vi "ER2007 Test Panel Mock Up.vi"() -> ()   [LabVIEW 2013]
uses:
  Controls/Global ER2007.vi
panel:
  in  "Defeated":bool
  in  "Sim":bool
  in  "Radio Cell Selects":T1(ring)
  out "Clock":string
  in  "Reset DAQ":bool
  out "VPA Err":bool
  out "Elap-T":string="Lapsed Hrs"
  out "Last-T":string="Time"
  out "ProdVol":string="Produced Vol (cc)"
  out "Dnstrm-P":string="Downstrm P (psi)"
  out "Delta-P":string="Delta-P (psi)"
  out "Pore-P":string="Pore P (psi)"
  out "Conf-P":string="Confining P (psi)"
  out "TB":string="T-B (°C)"
  out "TA":string="T-A (°C)"
  out "FF23":string="FF 2-3"
  out "ER23":string="E-R 2-3 (Ohm-m)"
  out "ER14":string="E-R 1-4 (Ohm-m)"
  out "ER13":string="E-R 1-3 (Ohm-m)"
  out "ER12":string="E-R 1-2 (Ohm-m)"
  out "SampID":string="Sample ID"
  out "Frequency":string="Frequency (Hz)"
  out "Status":string="Status"
  out "Other PC Busy":bool
  out "GCD Reset":bool
  in  "TakePt":bool
  out "System Error":bool
  out "Refresh":bool
  out "SetupCell":i32
  out "GCDCell":i32
  out "SelCell":i32
  out "C5-Status":bool caption="VPA"
  out "C4-Status":bool caption="Manual"
  out "C3-Status":bool caption="VPA"
  out "C2-Status":bool caption="Manual"
  out "C1-Status":bool caption="Manual"
  in  "GCD Progress Titles":string="Initialize  Main Eng  Determ-R  Final Vals Close HP Close NAII"
  out "GCD Prog":bool[](array[boolean])
  out "Selected Data Cell":i32
  out "Cell Data Idx":i32
  out "Cur Time":dbl
  out "Schd Times":dbl[](array[numeric])
  out "GCD Err":bool
  out "GCD Busy":bool
  out "A/D Err":bool
  out "DAQ Run":bool
  in  "Utilities":bool
  out "F 2-3":dbl[](array[numeric])=[6.3872, 0.0, 5.0918, 5.4196, 0.0, 5.8365, 5.8365, 0.0] format="%.2f"
  out "Cell":string[](array[string])=["200", "2000", "20000", "200000", "2000000", "Cell 6B", "6B", "6C"]
  out "Copyrightl":string="Program ER2005, Version 1.00, DCI Inc, Copyright 2005, All Rights Reserved"
  in  "CurVals":bool
  in  "History":bool
  in  "Setup":bool
  in  "Stop":bool
  out "ER 2-3":dbl[](array[numeric])=[6.3872, 0.0, 5.0918, 5.4196, 0.0, 5.8365, 5.8365, 0.0] format="%.3f"
  out "ER 1-4":dbl[](array[numeric])=[6.1683, 0.0, 5.0447, 5.2485, 0.0, 5.6703, 5.6703, 0.0] format="%.3f"
  out "ER 1-3":dbl[](array[numeric])=[6.0887, 0.0, 4.9169, 5.2753, 0.0, 5.5338, 5.5338, 0.0] format="%.3f"
  out "ER 1-2":dbl[](array[numeric])=[6.7304, 0.0, 5.356, 5.9831, 0.0, 6.0646, 6.0646, 0.0] format="%.3f"
  out "Status":bool[](array[boolean])=[FALSE, FALSE, FALSE, FALSE, FALSE, FALSE, TRUE, FALSE]
  # "Test Data"
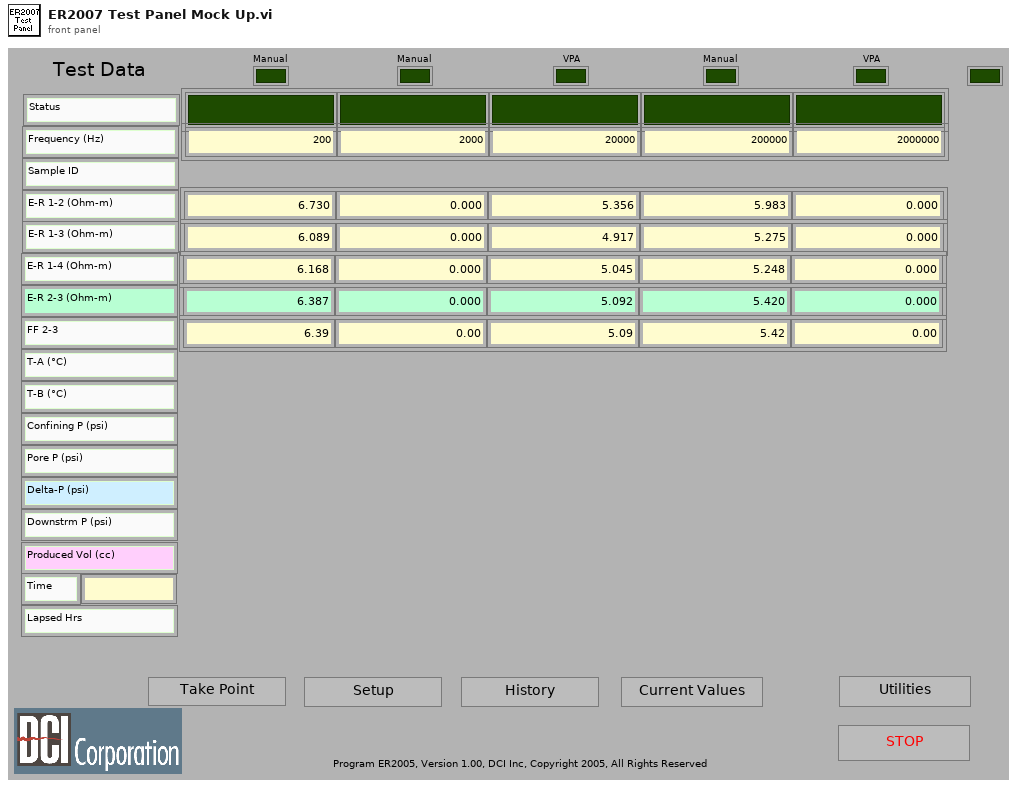
[diagram p1: front panel]
types:
  T1 = enum32{"No Selection", "CS 1", "CS 2", "CS 3", "CS 4", "CS 5", "CS 6"}
  T2 = cluster{"PageTitle":string, "NumLines":i32, "ChlNum":string[], "ChlDesc":string[], "ChlUnits":string[], "ChlZero":sgl[], "ChlFactor":sgl[], "ChlConfig":u16[]}[]
  T3 = enum16{"Cell 1", "Cell 2", "Cell 3", "Cell 4", "Cell 5", "Cell 6A", "Cell 6B", "Cell 6C"}[]
  T4 = cluster{"CurCell":i32, "Cell Data":cluster{"Cell ID":i32, "Cell Status":enum16{"Inactive", "Setup", "Active", "Done"}, "Project":string, "Sample #":string, "Rock Type":string, "Fluid Pair":string, "Rw":dbl, "Rw Temp":dbl, "Length":dbl, "Diameter":dbl, "Porosity":dbl, "Permeability":dbl, "4P":bool, "ElectSpace":dbl, "Frequency":dbl, "Amplitude":dbl, "DAQ Period":u32, "DAQ Units":u16, "Start Time":dbl, "Next Time":dbl, "Datafile":path, "Last Pore Vol":dbl, "Last Pore Xdcr":enum16{"<none>", "Lo Range", "Hi Range"}, "Last Resistor":enum16{"<none>", "Resistor 1", "Resistor 2", "Resistor 3", "Resistor 4", "Resistor 5", "Resistor 6"}, "CurData":dbl[][], "Comment":string}[]}
  T5 = cluster{"Cell ID":i32, "Cell Status":enum16{"Inactive", "Setup", "Active", "Done"}, "Project":string, "Sample #":string, "Rock Type":string, "Fluid Pair":string, "Rw":dbl, "Rw Temp":dbl, "Length":dbl, "Diameter":dbl, "Porosity":dbl, "Permeability":dbl, "4P":bool, "ElectSpace":dbl, "Frequency":dbl, "Amplitude":dbl, "DAQ Period":u32, "DAQ Units":u16, "Start Time":dbl, "Next Time":dbl, "Datafile":path, "Last Pore Vol":dbl, "Last Pore Xdcr":enum16{"<none>", "Lo Range", "Hi Range"}, "Last Resistor":enum16{"<none>", "Resistor 1", "Resistor 2", "Resistor 3", "Resistor 4", "Resistor 5", "Resistor 6"}, "CurData":dbl[][], "Comment":string}[]
  T6 = cluster{"Cell ID":i32, "Cell Status":enum16{"Inactive", "Setup", "Active", "Done"}, "Project":string, "Sample #":string, "Rock Type":string, "Fluid Pair":string, "Rw":dbl, "Rw Temp":dbl, "Length":dbl, "Diameter":dbl, "Porosity":dbl, "Permeability":dbl, "4P":bool, "ElectSpace":dbl, "Frequency":dbl, "Amplitude":dbl, "DAQ Period":u32, "DAQ Units":u16, "Start Time":dbl, "Next Time":dbl, "Datafile":path, "Last Pore Vol":dbl, "Last Pore Xdcr":enum16{"<none>", "Lo Range", "Hi Range"}, "Last Resistor":enum16{"<none>", "Resistor 1", "Resistor 2", "Resistor 3", "Resistor 4", "Resistor 5", "Resistor 6"}, "CurData":dbl[][], "Comment":string}
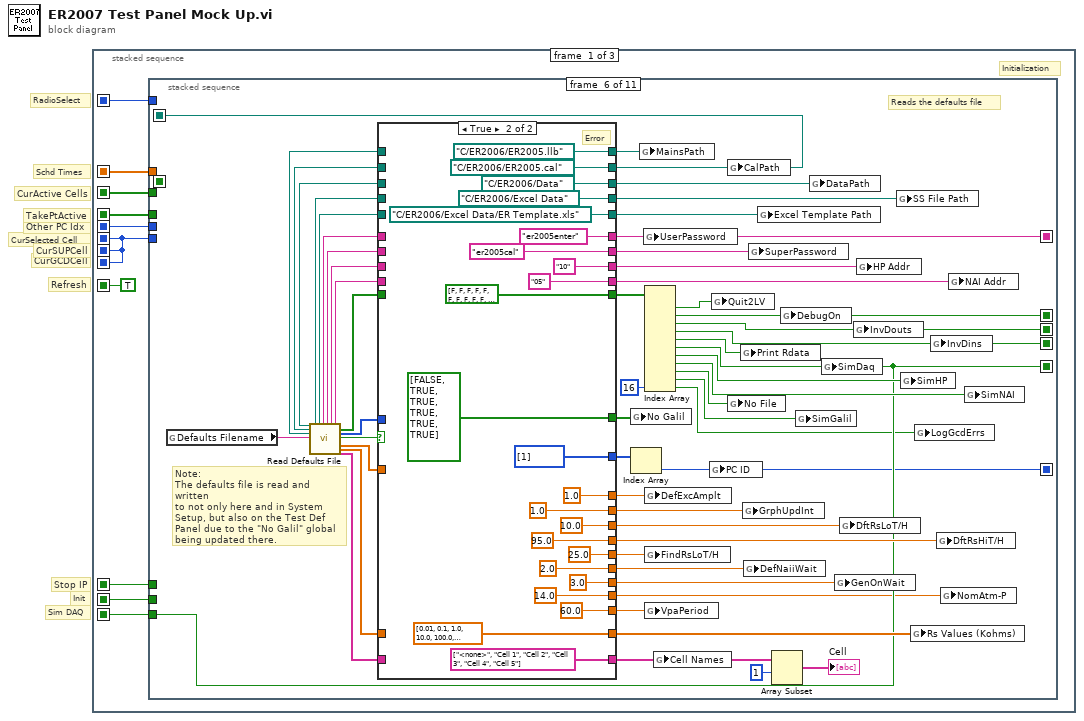
[diagram p0: block diagram]
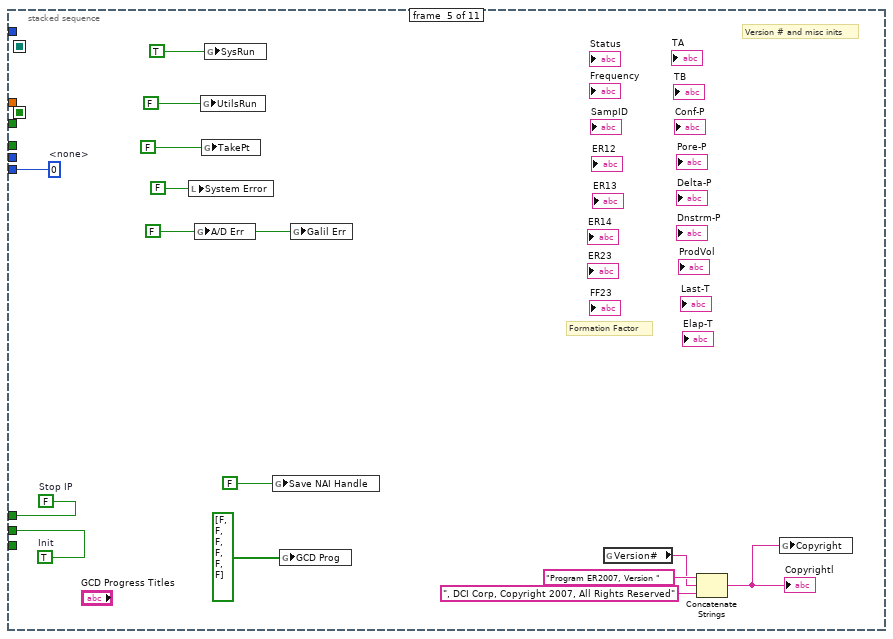
[diagram p6: hidden frame]
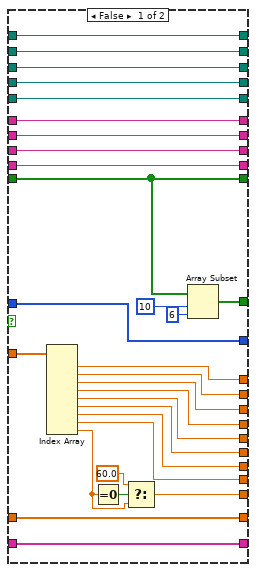
[diagram p7: hidden frame]
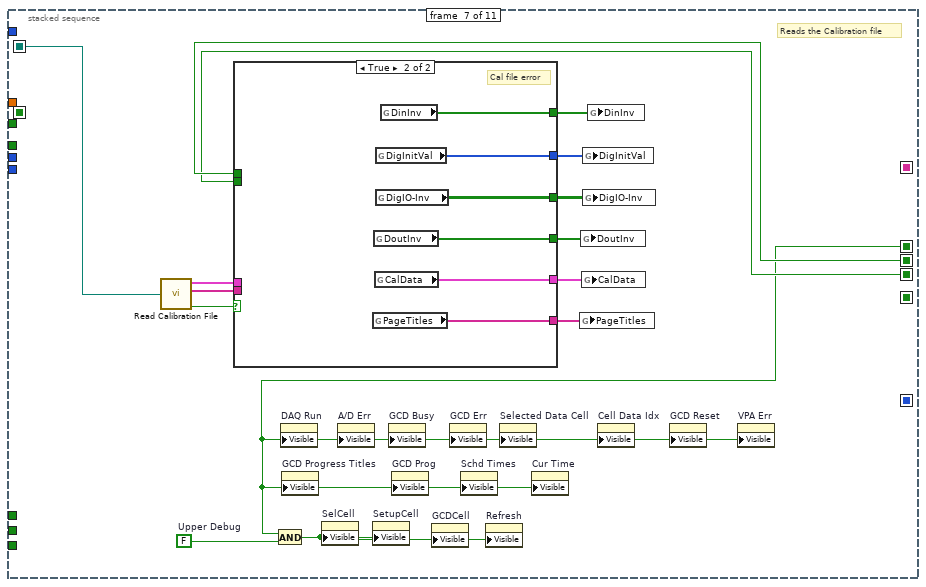
[diagram p8: hidden frame]
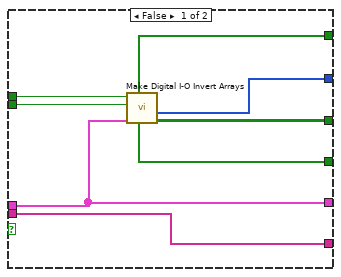
[diagram p9: hidden frame]
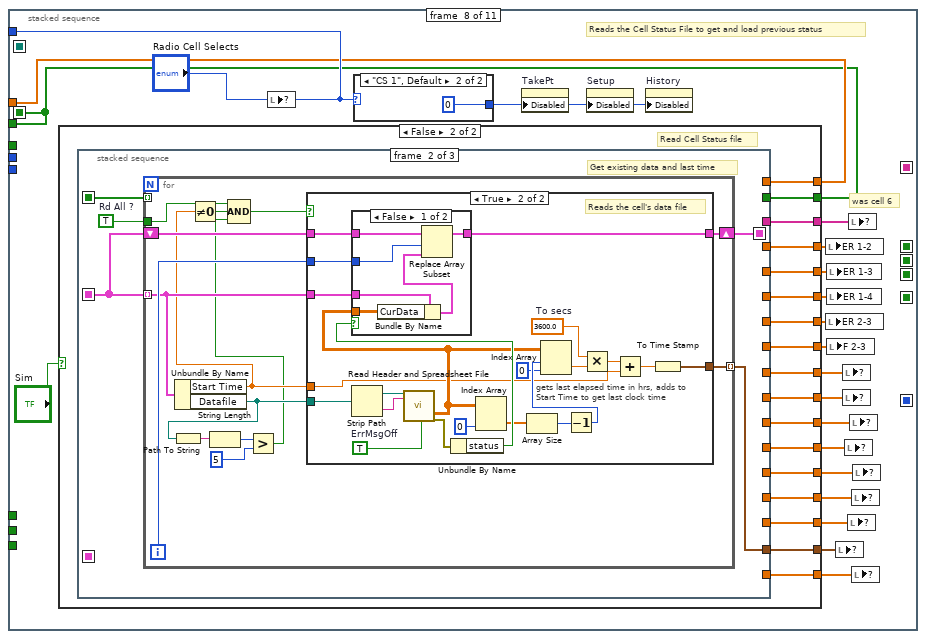
[diagram p10: hidden frame]
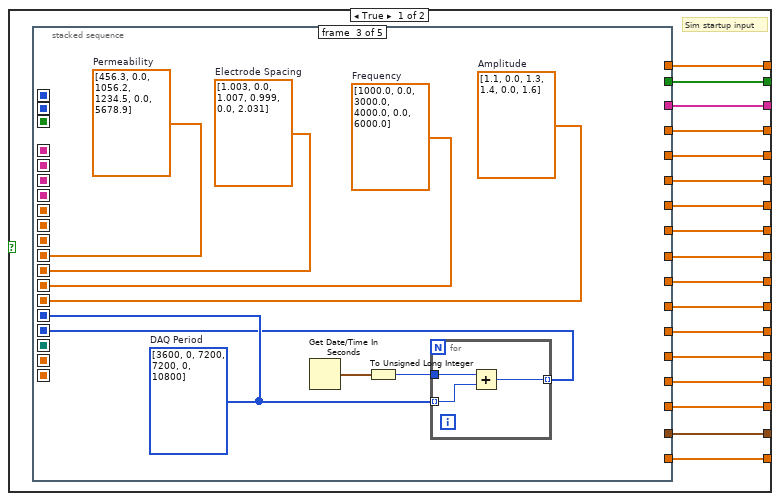
[diagram p11: hidden frame]
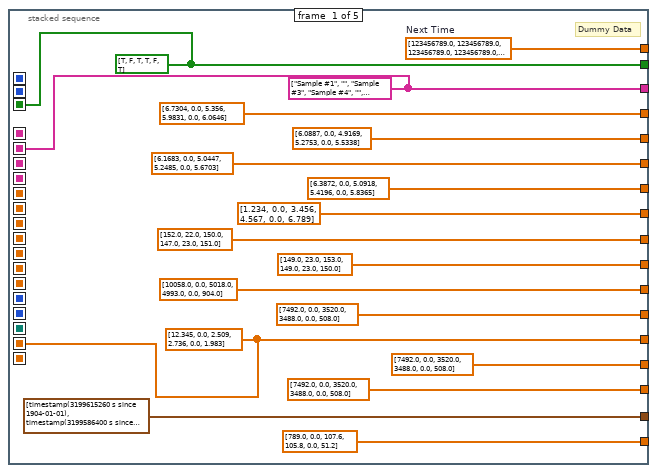
[diagram p12: hidden frame]
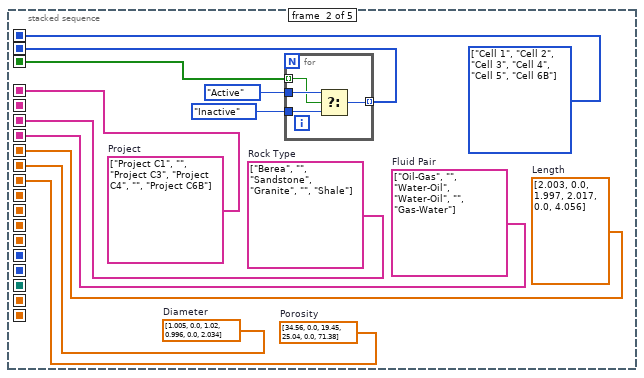
[diagram p13: hidden frame]
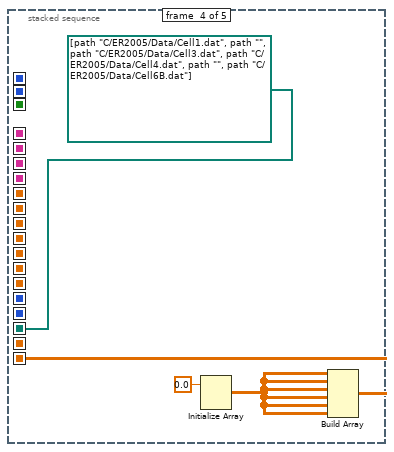
[diagram p14: hidden frame]
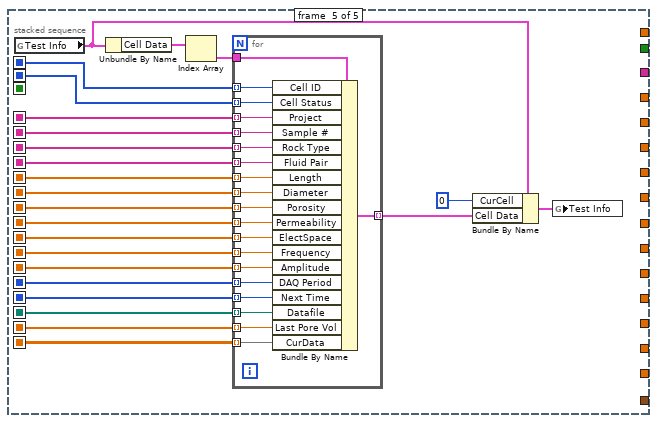
[diagram p15: hidden frame]
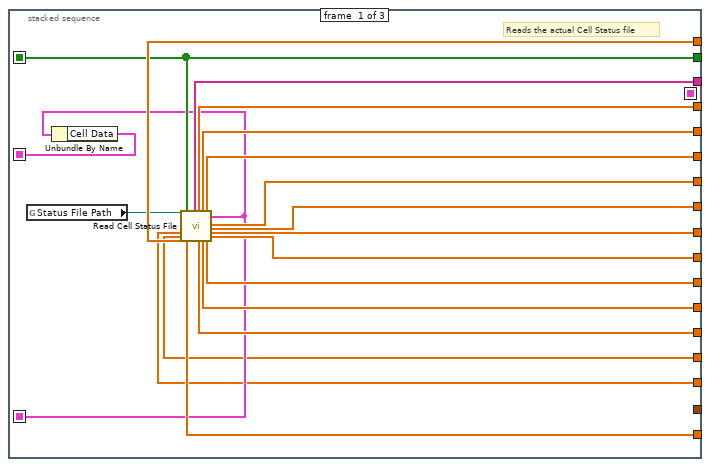
[diagram p16: hidden frame]
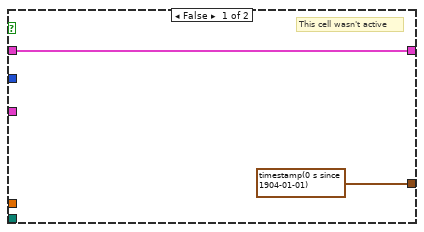
[diagram p17: hidden frame]
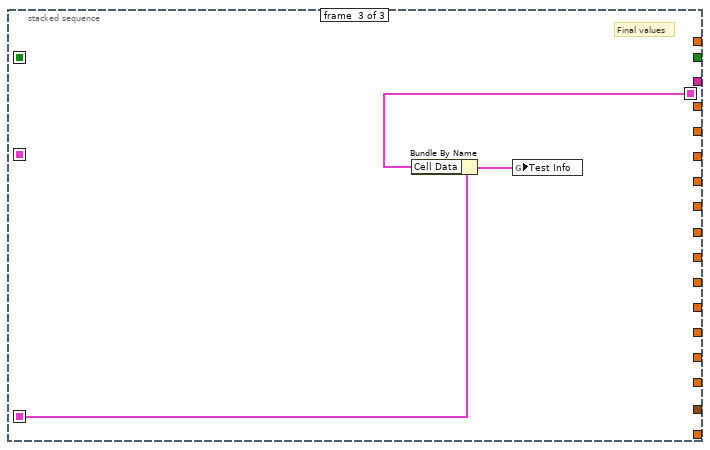
[diagram p19: hidden frame]
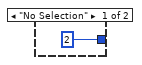
[diagram p20: hidden frame]
diagram:
  # "Sim DAQ"
  # "Init"
  # "Stop IP"
  # "Refresh"
  # "CurGCDCell"
  # "CurSUPCell"
  # "CurSelected Cell"
  # "Other PC Idx"
  # "TakePtActive"
  # "CurActive Cells"
  # "Schd Times"
  # "RadioSelect"
  n1 = stacked-sequence {
    seq-local: [w10 _ _] -> [_ w451 _]
    seq-local: [w9 _ _] -> [_ w450 _]
    seq-local: [w8 _ _] -> [_ w449 _]
    seq-local: [w7 _ _] -> [_ w448 _]
    seq-local: [w6 _ _] -> [_ w447 _]
    seq-local: [w5 _ _] -> [_ w445 _]
    seq-local: [w5 _ _] -> [_ w446 _]
    seq-local: [w5 _ _] -> [_ w444 _]
    seq-local: [TRUE _ _] -> [_ w443 _]
    seq-local: [w3 _ _] -> [_ w442 w1325]
    seq-local: [w2 _ _] -> [_ w441 _]
    seq-local: [w1 _ _] -> [_ w440 _]
    frame #0 {
      # "Initialization"
      n2 = stacked-sequence {
        seq-local: [_ _ _ _ _ w58 _ _ _ _ _] -> [_ _ _ _ _ _ w140 _ _ _ _]
        seq-local: [_ _ _ _ _ w57 _ _ _ _ _] -> [_ _ _ _ _ _ _ _ _ _ _]
        seq-local: [_ _ _ _ _ w52 _ _ _ _ _] -> [_ _ _ _ _ _ w142 _ _ _ _]
        seq-local: [_ _ _ _ _ w53 _ _ _ _ _] -> [_ _ _ _ _ _ w141 _ _ _ _]
        seq-local: [_ _ _ _ _ _ _ w162 _ _ _] -> [_ _ _ _ _ _ _ _ _ w391 _]
        seq-local: [_ _ _ _ _ w50 _ _ _ _ _] -> [_ _ _ _ _ _ w131 _ _ _ _]
        seq-local: [_ _ _ _ _ w35 _ _ _ _ _] -> [_ _ _ _ _ _ _ _ w383 _ _]
        seq-local: [_ _ _ _ _ w34 _ _ _ _ _] -> [_ _ _ _ _ _ _ _ w380 _ _]
        tunnel: [_ _ _ _ _ _ _ w164 _ _ _] -> w10
        tunnel: [_ _ _ _ _ _ _ "Radio Cell Selects" _ _ _] -> w9
        tunnel: [_ _ _ _ w22 _ _ _ _ _ _] -> w8
        tunnel: [_ _ _ _ _ _ _ w162 _ _ _] -> w7
        tunnel: [_ _ _ _ _ _ _ _ _ w388 _] -> w6
        tunnel: [_ _ _ _ w13 _ _ _ _ _ _] -> w5
        tunnel: [_ _ _ _ _ w35 _ _ _ _ _] -> w3
        tunnel: [_ _ _ _ _ _ _ _ w379 _ _] -> w2
        tunnel: [_ _ _ _ w11 _ _ _ _ _ _] -> w1
        frame #0 {
          # "VERSION                                             DESCRIPTION                                                           DATE \n------- --------------------------------------------------------------------------------------------------------------- --------\n  1.00  Original release                                                                                                 06/2007\n  1.10  Front Pnl clock; Are You Sure exit; History Table date & time; dat file comments; calc fail repeat; brine calc   10/2007\n        mods\n  1.11  CFJ Field mod\n  1.12  2P/4P on Test Setup always ungrayed; History Panel: export to Excel fix, remembers graph scales, auto scroll to   5/2008\n        bottom of table; \"VpaPeriod\" added to defaults file, Sys Setup and DAQ loop;"
          # "Version Documentation"
        }
        frame #1 {
          # "New Cell Status Format\n\n[GenInfo]\nTitle=\"Cell Status Data File\"\nVersion=1.00\nLast Write=8/7/2005\nCurCell=\"2\"\n*NumCells=\"5\"\n[Cell 1 Status]\nCell ID=\"Cell 1\"\nStatus=Inactive\nProject=\"Project Cell 1\"\nSample ID=\"Sample #1\"\nRock Type=Granite\nFluid Pair=\"Brine & Air\"\nRw=11.000000\nRw Temp=22.000000\nLength=5.080000\nDiameter=2.540000\nPorosity=33.000000\nPermeability=8.000000\n2P/4P=4P\nElect Spacing=2.540000\nFrequency=1000.000000\nAmplitude=1.000000\nDAQ Period=1\nDAQ Units=Hrs\nStart Time=3205931570.670000\nNext Time=3205935200.670000\nFilename=\"C:\\\\ER2005\\\\Data\\\\Cell 1 Data.dat\"\nPore Volume=1.000000\n*Pore Transducer=\"Lo Range\"\nLast Resistor=\"Resistor 5\"\nER 1-2=4023.631104\nER 1-3=2923.760010\nER 1-4=3594.040039\nER 2-3=2434.518066\nFF 2-3=235.399994\nTemp A=24.799999\nTemp B=24.799999\nConf Press=5.000000\nPore Press=2.330000\nDelta-Press=\nPore-Down=\n[Cell 2 Status]"
          # "New Data File Format-Data Line\n\n                        Reals\nCol #  Process Variable Col #\n----- ----------------- -----\n  1   Point Flag\n  2   Point Date\n  3   Point Time\n  4   Elapsed Time (hrs)   1\n  5   ER 1-2               2\n  6   ER 1-3               3\n  7   ER 1-4               4\n  8   ER 2-3               5\n  9   F 2-3                6\n 10   T-A                  7\n 11   T-B                  8\n 12   Conf P (ER2005 NOP)  9\n 13   Pore P (ER2005 Pc)  10\n 14   Delta-P             11\n 15   Downstrm P (Pc-d)   12\n 16   Produced Vol        13\n 17   C14                 14\n 18   C23                 15\n 19   Comment"
          # "Dynamically Launched vi's:                     Other Required Files: simply copy them to System32\n-----------------------------------------      --------------------------------------------------------\nER2007 Are You Sure Popup Panel.vi             C:\\Windows\\System32\\instrsup.dll - used by NAII vi's\nER2007 Background DAQ Loop.vi                  C:\\Windows\\System32\\NAI2250.dll - used by NAII vi's\nER2007 Calibration Panel.vi                    C:\\Windows\\System32\\DMC32.dll - used by Galil vi's\nER2007 Current Values Panel.vi                 \nER2007 Data History Panel.vi\nER2007 Get Cell Data.vi\nER2007 Maintenance Panel.vi\nER2007 Password Popup Panel.vi\nER2007 System Setup Panel.vi\nER2007 Take Data Popup Panel.vi\nER2007 Test Definition Panel.vi\nER2007 Utilities Menu Panel.vi\nC:\\Program Files\\National Instruments\\LabVIEW 7.1\\vi.lib\\\n (cont)  addons\\_office\\_exclsub.llb\\_Excel Dynamic VIs.vi"
          # "Data File Format-Header\n\nStart Date\nStart Time\nFilename\nProject\nSample ID\nRock Type\nFluid Pair\nRw\nRt\nFrequency\nAmplitude\nDAQ Period (mins)\nLength\nDiameter\nPorosity\nPermeability\nElectrode Spacing"
          # "The arrays and controls on the front panel are a Arial Bold at 20 pt (18 pt plus two cntrl+)\nThe front panel color (matches Logo): Hue-135; Sat-43; Lum-109; Red-95; Grn-121; Blue-137"
          # "Notes and misc initilization"
        }
        frame #2 {
          # "More notes: Device 1 hardware assignments"
          # "PCI-6220 PV Assignments\n\n                      Connector 0\n        DIGITAL OUTS                ANALOG INS\n----------------------------  ------------------------\nP0.0    Shunt NOP1/Pc1A       AI 0    NOP1\nP0.1    SCL1                  AI 1    TC1A\nP0.2    SCL2                  AI 2    TC1B\nP0.3    Shunt Pc1B            AI 3    Pc1B\nP0.4    Auto Enable           AI 4    <spare>\nP0.5    RSCL1                 AI 5    <spare>\nP0.6    <spare>               AI 6    <spare>\nP0.7    RSCL2                 AI 7    <spare>\n\nP1.0    RSCL3                 AI 8    Pc1A\nP1.1    YCL1                  AI 9    CJ1A\nP1.2    YCL2                  AI 10   CJ1B\nP1.3    YCL3                  AI 11   <spare>\nP1.4    YCL4                  AI 12   <spare>\nP1.5    <spare>               AI 13   <spare>\nP1.6    Lockout               AI 14   <spare>\nP1.7    <spare>               AI 15   <spare>\n\n        DIGITAL INS\n----------------------------\nP2.0    <spare>\nP2.1    <spare>\nP2.2    <spare>\nP2.3    <spare>\nP2.4    <spare>\nP2.5    <spare>\nP2.6    <spare>\nP2.7    <spare>"
        }
        frame #3 {
          # "GPIB Setup and Operational Notes\n\n1) Using MAX, setup the PC #1 GPIB board as System\n   Controller with a primary address of 1.  Setup the\n   PC #2 GBIP board as a Non-System Controller with a\n   primary address of 2.\n2) Initialization is still a problem\n3) When PC #1 is active (taking a point), it asserts\n   Send IFC to clear the bus and take charge.  After\n   it has completed, it returns CIC control to PC #2\n   using PassControl."
          # "PCI-6224 PV Assignments By Connector Number\n\n                      Connector 1\n        DIGITAL OUTS                ANALOG INS\n----------------------------  ------------------------\nP0.8    Shunt NOP4/Pc4A       AI 16   NOP4\nP0.9    <spare>               AI 17   TC4A\nP0.10   <spare>               AI 18   TC4B\nP0.11   Shunt NOP5/Pc4B       AI 19   Pc4B\nP0.12   <spare>               AI 20   <spare>\nP0.13   Shunt Pc5A/Pc5B       AI 21   Pc5A\nP0.14   <spare>               AI 22   TC5A\nP0.15   <spare>               AI 23   TC5B\n\n                              AI 24   Pc4A\n                              AI 25   CJ4A\n                              AI 26   CJ4B\n                              AI 27   NOP5\n                              AI 28   <spare>\n                              AI 29   Pc5B\n                              AI 30   CJ5A\n                              AI 31   CJ5B"
          # "PCI-6224 PV Assignments By Connector Number\n\n                      Connector 0\n        DIGITAL OUTS                ANALOG INS\n----------------------------  ------------------------\nP0.0    Shunt NOP2/Pc2A       AI 0    NOP2\nP0.1    <spare>               AI 1    TC2A\nP0.2    <spare>               AI 2    TC2B\nP0.3    Shunt NOP3/Pc2B       AI 3    Pc2B\nP0.4    <spare>               AI 4    <spare>\nP0.5    Shunt Pc3A/Pc3B       AI 5    Pc3A\nP0.6    <spare>               AI 6    TC3A\nP0.7    <spare>               AI 7    TC3B\n\nP1.0    <spare>               AI 8    Pc2A\nP1.1    <spare>               AI 9    CJ2A\nP1.2    <spare>               AI 10   CJ2B\nP1.3    <spare>               AI 11   NOP3\nP1.4    <spare>               AI 12   <spare>\nP1.5    <spare>               AI 13   Pc3A\nP1.6    <spare>               AI 14   CJ3A\nP1.7    <spare>               AI 15   CJ3B\n\n        DIGITAL INS\n----------------------------\nP2.0    Busy 1\nP2.1    Busy 2\nP2.2    <spare>\nP2.3    <spare>\nP2.4    <spare>\nP2.5    <spare>\nP2.6    <spare>\nP2.7    <spare>"
          # "More notes: Device 2 hardware assignments"
        }
        frame #4 {
          w11 = FALSE  # Stop IP
          w12 = FALSE ("A/D Err")
          w13 = 0  # <none>
          w22 = TRUE  # Init
          # "Formation Factor"
          # "Version # and misc inits"
          n3 = local write "System Error"(FALSE ("System Error")) -> ()
          n4 = global write "Global ER2007.vi" "A/D Err"(w12) -> ()
          n5 = global write "Global ER2007.vi" "UtilsRun"(FALSE ("UtilsRun")) -> ()
          n6 = global write "Global ER2007.vi" "TakePt"(FALSE ("New Setup")) -> ()
          n7 = global write "Global ER2007.vi" "SysRun"(TRUE ("SysRun")) -> ()
          n8 = global write "Global ER2007.vi" "Save NAI Handle"(FALSE ("Save NAI Handle")) -> ()
          n9 = global write "Global ER2007.vi" "GCD Prog"(bool[] [FALSE, FALSE, FALSE, FALSE, FALSE, FALSE] ("GCD Prog")) -> ()
          n10 = global write "Global ER2007.vi" "Galil Err"(w12) -> ()
          n11 = global read "Global ER2007.vi" "Version#"() -> (w20:string)
          n12 = Concatenate Strings("Program ER2007, Version " ("Substring"), w20, ", DCI Corp, Copyright 2007, All Rights Reserved" ("Substring")) -> (w19:string)
          "Copyrightl" <- w19
          n13 = global write "Global ER2007.vi" "Copyright"(w19) -> ()
        }
        frame #5 {
          # "Note:\nThe defaults file is read and written\nto not only here and in System\nSetup, but also on the Test Def\nPanel due to the \"No Galil\" global\nbeing updated there."
          # "Reads the defaults file"
          n14 = global read "Global ER2007.vi" "Defaults Filename"() -> (w37:string)
          n15 = call "Read Defaults File.vi"("Filename"=w37) -> ("DirPath3"=w73:path, "DirPath2"=w74:path, "DirPath1"=w75:path, "DirPath4"=w66:path, "DirPath5"=w65:path, "String1"=w72:string, "String2"=w71:string, "String3"=w69:string, "String4"=w68:string, "BooleanArray"=w77:bool[], "IntegerArray1"=w64:i32[], "ErrOut"=w78:bool, "RealArray1"=w70:dbl[], "RealArray2"=w67:dbl[], "StringArray"=w36:string[])  [unwired: 12 out]
          n16 = case shown="True" w78 {
            tunnel: w77 -> [w86 _]
            tunnel: [w86 bool[] [FALSE, FALSE, FALSE, FALSE, FALSE, FALSE, FALSE, FALSE, FALSE, FALSE, FALSE, FALSE] ("BooleanArray")] -> w76
            tunnel: [w107 path "C:/ER2006/ER2005.llb" ("DirPath1")] -> w59
            tunnel: w75 -> [w107 _]
            tunnel: [w106 path "C:/ER2006/ER2005.cal" ("DirPath2")] -> w58
            tunnel: w74 -> [w106 _]
            tunnel: [w105 path "C:/ER2006/Data" ("DirPath3")] -> w62
            tunnel: w73 -> [w105 _]
            tunnel: [w104 "er2005enter" ("String1")] -> w57
            tunnel: w72 -> [w104 _]
            tunnel: [w103 "er2005cal" ("String2")] -> w56
            tunnel: w71 -> [w103 _]
            tunnel: w70 -> [w100 _]
            tunnel: [w102 "10" ("String3")] -> w55
            tunnel: w69 -> [w102 _]
            tunnel: [w101 "05" ("String4")] -> w54
            tunnel: w68 -> [w101 _]
            tunnel: [w99 1.0] -> w45
            tunnel: [w98 1.0] -> w44
            tunnel: [w97 10.0] -> w43
            tunnel: [w96 95.0] -> w42
            tunnel: w67 -> [w95 _]
            tunnel: [w95 dbl[] [0.01, 0.1, 1.0, 10.0, 100.0, 1000.0] ("RealArray2")] -> w38
            tunnel: [w94 25.0] -> w41
            tunnel: [w93 path "C:/ER2006/Excel Data" ("SS File Path")] -> w61
            tunnel: w66 -> [w93 _]
            tunnel: [w92 2.0] -> w40
            tunnel: [w91 3.0] -> w39
            tunnel: [w90 path "C:/ER2006/Excel Data/ER Template.xls" ("Excel Template Path")] -> w60
            tunnel: w65 -> [w90 _]
            tunnel: w64 -> [w89 _]
            tunnel: [w89 i32[] [1] ("IntegerArray1")] -> w63
            tunnel: w36 -> [w88 _]
            tunnel: [w88 string[] ["<none>", "Cell 1", "Cell 2", "Cell 3", "Cell 4", "Cell 5"] ("StringArray")] -> w31
            tunnel: [w87 14.0 ("NomAtm-P")] -> w32
            tunnel: [w83 bool[] [FALSE, TRUE, TRUE, TRUE, TRUE, TRUE]] -> w28
            tunnel: [w79 60.0 ("VpaPeriod")] -> w25
            frame False {
              n17 = Index Array(array=w100) -> (element #1=w99:dbl, element #2=w98:dbl, element #3=w97:dbl, element #4=w96:dbl, element #5=w94:dbl, element #6=w92:dbl, element #7=w91:dbl, element #8=w87:dbl, element #9=w80:dbl)  [unwired: 9 in]
              n18 = Equal To 0?(x=w80) -> (x = 0?=w82:bool)
              n19 = Select(t=60.0, s=w82, f=w80) -> (s? t:f=w79:dbl)
              n20 = Array Subset(array=w86, index=10, length=6) -> (w83:bool[])
            }
            frame True {
              # "Error"
            }
          }
          n21 = global write "Global ER2007.vi" "No Galil"(w28) -> ()
          n22 = Index Array(array=w63) -> (element=w34:i32)  [unwired: 1 in]
          n23 = global write "Global ER2007.vi" "MainsPath"(w59) -> ()
          n24 = global write "Global ER2007.vi" "UserPassword"(w57) -> ()
          n25 = Index Array(array=w76, index #11=16 ("index")) -> (element #1=w51:bool, element #2=w50:bool, element #3=w52:bool, element #4=w53:bool, element #5=w49:bool, element #6=w35:bool, element #7=w48:bool, element #8=w47:bool, element #9=w46:bool, element #10=w33:bool, element #11=w26:bool)  [unwired: 10 in]
          n26 = global write "Global ER2007.vi" "DefExcAmplt"(w45) -> ()
          n27 = global write "Global ER2007.vi" "FindRsLoT/H"(w41) -> ()
          n28 = global write "Global ER2007.vi" "VpaPeriod"(w25) -> ()
          n29 = global write "Global ER2007.vi" "Cell Names"(w31) -> ()
          n30 = global write "Global ER2007.vi" "PC ID"(w34) -> ()
          n31 = global write "Global ER2007.vi" "Quit2LV"(w51) -> ()
          n32 = global write "Global ER2007.vi" "CalPath"(w58) -> ()
          n33 = global write "Global ER2007.vi" "No File"(w46) -> ()
          n34 = global write "Global ER2007.vi" "Print Rdata"(w49) -> ()
          n35 = global write "Global ER2007.vi" "GrphUpdInt"(w44) -> ()
          n36 = global write "Global ER2007.vi" "DefNaiiWait"(w40) -> ()
          n37 = global write "Global ER2007.vi" "SuperPassword"(w56) -> ()
          n38 = global write "Global ER2007.vi" "Excel Template Path"(w60) -> ()
          n39 = Array Subset(array=w31, index=1) -> (→"Cell":string[])  [unwired: 1 in]
          n40 = global write "Global ER2007.vi" "DebugOn"(w50) -> ()
          n41 = global write "Global ER2007.vi" "SimGalil"(w33) -> ()
          n42 = global write "Global ER2007.vi" "DataPath"(w62) -> ()
          n43 = global write "Global ER2007.vi" "SimDaq"(w35) -> ()
          n44 = global write "Global ER2007.vi" "GenOnWait"(w39) -> ()
          n45 = global write "Global ER2007.vi" "DftRsLoT/H"(w43) -> ()
          n46 = global write "Global ER2007.vi" "InvDouts"(w52) -> ()
          n47 = global write "Global ER2007.vi" "HP Addr"(w55) -> ()
          n48 = global write "Global ER2007.vi" "SS File Path"(w61) -> ()
          n49 = global write "Global ER2007.vi" "SimHP"(w48) -> ()
          n50 = global write "Global ER2007.vi" "Rs Values (Kohms)"(w38) -> ()
          n51 = global write "Global ER2007.vi" "LogGcdErrs"(w26) -> ()
          n52 = global write "Global ER2007.vi" "InvDins"(w53) -> ()
          n53 = global write "Global ER2007.vi" "DftRsHiT/H"(w42) -> ()
          n54 = global write "Global ER2007.vi" "NomAtm-P"(w32) -> ()
          n55 = global write "Global ER2007.vi" "NAI Addr"(w54) -> ()
          n56 = global write "Global ER2007.vi" "SimNAI"(w47) -> ()
        }
        frame #6 {
          w138 = FALSE  # Upper Debug
          # "Reads the Calibration file"
          n57 = call "Read Calibration File.vi"("Filepath"=w140) -> ("CalData"=w144:T2, "PageTitles"=w143:string[], "ErrOut"=w145:bool)  [unwired: 1 in, 2 out]
          n58 = case shown="True" w145 {
            tunnel: w144 -> [w152 _]
            tunnel: w143 -> [w153 _]
            tunnel: [w152 w154] -> w133
            tunnel: [w153 w155] -> w132
            tunnel: w142 -> [w151 _]
            tunnel: w141 -> [w150 _]
            tunnel: [w149 w156] -> w134
            tunnel: [w148 w157] -> w135
            tunnel: [w147 w158] -> w136
            tunnel: [w146 w159] -> w137
            frame False {
              n59 = call "Make Digital I-O Invert Arrays.vi"("CalDataIn"=w152, "InvDins"=w150, "InvDouts"=w151) -> ("DIO-Inv"=w148:bool[][], "DoutInit"=w147:i32[], "DoutInv (1D)"=w149:bool[], "DinInv (1D)"=w146:bool[])  [unwired: 1 in, 4 out]
            }
            frame True {
              # "Cal file error"
              n60 = global read "Global ER2007.vi" "PageTitles"() -> (w155:string[])
              n61 = global read "Global ER2007.vi" "DoutInv"() -> (w156:bool[])
              n62 = global read "Global ER2007.vi" "CalData"() -> (w154:T2)
              n63 = global read "Global ER2007.vi" "DigInitVal"() -> (w158:i32[])
              n64 = global read "Global ER2007.vi" "DigIO-Inv"() -> (w157:bool[][])
              n65 = global read "Global ER2007.vi" "DinInv"() -> (w159:bool[])
            }
          }
          n66 = And(x=w131, y=w138) -> (x .and. y?=w139:bool)
          n67 = property on="DAQ Run" class="Bool (strict)"("Visible"=w131) -> ()  [unwired: 2 in, 2 out]
          n68 = property on="GCD Progress Titles" class="Str"("Visible"=w131) -> ()  [unwired: 2 in, 2 out]
          n69 = property on="SelCell" class="DigNum (strict)"("Visible"=w139) -> ()  [unwired: 2 in, 2 out]
          n70 = property on="A/D Err" class="Bool (strict)"("Visible"=w131) -> ()  [unwired: 2 in, 2 out]
          n71 = property on="SetupCell" class="DigNum (strict)"("Visible"=w139) -> ()  [unwired: 2 in, 2 out]
          n72 = property on="GCD Busy" class="Bool (strict)"("Visible"=w131) -> ()  [unwired: 2 in, 2 out]
          n73 = property on="GCD Prog" class="Arr (strict)"("Visible"=w131) -> ()  [unwired: 2 in, 2 out]
          n74 = property on="GCDCell" class="DigNum (strict)"("Visible"=w139) -> ()  [unwired: 2 in, 2 out]
          n75 = property on="GCD Err" class="Bool (strict)"("Visible"=w131) -> ()  [unwired: 2 in, 2 out]
          n76 = property on="Schd Times" class="Arr (strict)"("Visible"=w131) -> ()  [unwired: 2 in, 2 out]
          n77 = property on="Refresh" class="Bool (strict)"("Visible"=w139) -> ()  [unwired: 2 in, 2 out]
          n78 = property on="Selected Data Cell" class="DigNum (strict)"("Visible"=w131) -> ()  [unwired: 2 in, 2 out]
          n79 = property on="Cur Time" class="DigNum (strict)"("Visible"=w131) -> ()  [unwired: 2 in, 2 out]
          n80 = global write "Global ER2007.vi" "PageTitles"(w132) -> ()
          n81 = global write "Global ER2007.vi" "DoutInv"(w134) -> ()
          n82 = global write "Global ER2007.vi" "CalData"(w133) -> ()
          n83 = global write "Global ER2007.vi" "DigInitVal"(w136) -> ()
          n84 = global write "Global ER2007.vi" "DigIO-Inv"(w135) -> ()
          n85 = global write "Global ER2007.vi" "DinInv"(w137) -> ()
          n86 = property on="Cell Data Idx" class="DigNum (strict)"("Visible"=w131) -> ()  [unwired: 2 in, 2 out]
          n87 = property on="GCD Reset" class="Bool (strict)"("Visible"=w131) -> ()  [unwired: 2 in, 2 out]
          n88 = property on="VPA Err" class="Bool (strict)"("Visible"=w131) -> ()  [unwired: 2 in, 2 out]
        }
        frame #7 {
          # "was cell 6"
          # "Reads the Cell Status File to get and load previous status"
          n89 = case shown="False" "Sim" {
            tunnel: [w196 w292] -> w162
            tunnel: [w195 w304] -> w176
            tunnel: [w194 w303] -> w175
            tunnel: [w193 w302] -> w174
            tunnel: [w192 w301] -> w173
            tunnel: [w191 w300] -> w172
            tunnel: [w190 w299] -> w171
            tunnel: [w189 w298] -> w170
            tunnel: [w188 w297] -> w169
            tunnel: [w187 w296] -> w168
            tunnel: [w186 w295] -> w167
            tunnel: [w185 w294] -> w166
            tunnel: [w184 w293] -> w165
            tunnel: [w183 w291] -> w164
            tunnel: [w182 w290] -> w163
            tunnel: [w181 w289] -> w161
            tunnel: [w180 w288] -> w160
            frame True {
              # "Sim startup input"
              n90 = stacked-sequence {
                seq-local: [_ _ w229 _ _] -> [_ _ _ _ w251]
                seq-local: [_ _ w230 _ _] -> [_ _ _ _ w252]
                seq-local: [w211 _ _ _ _] -> [_ _ _ _ w264]
                seq-local: [_ w217 _ _ _] -> [_ _ _ _ w261]
                seq-local: [_ w216 _ _ _] -> [_ _ _ _ w260]
                seq-local: [_ w215 _ _ _] -> [_ _ _ _ w259]
                seq-local: [_ w214 _ _ _] -> [_ _ _ _ w258]
                seq-local: [_ _ w236 _ _] -> [_ _ _ _ w257]
                seq-local: [_ _ w235 _ _] -> [_ _ _ _ w256]
                seq-local: [_ _ w234 _ _] -> [_ _ _ _ w255]
                seq-local: [_ _ w233 _ _] -> [_ _ _ _ w254]
                seq-local: [w213 _ _ _ _] -> [_ _ _ _ w253]
                seq-local: [w212 _ _ _ _] -> [_ w223 _ _ _]
                seq-local: [_ w224 _ _ _] -> [_ _ _ _ w267]
                seq-local: [_ w220 _ _ _] -> [_ _ _ _ w265]
                seq-local: [_ w219 _ _ _] -> [_ _ _ _ w263]
                seq-local: [_ w218 _ _ _] -> [_ _ _ _ w262]
                seq-local: [_ _ _ path[] [path "C:/ER2005/Data/Cell1.dat", path "", path "C:/ER2005/Data/Cell3.dat", path "C:/ER2005/Data/Cell4.dat", path "", path "C:/ER2005/Data/Cell6B.dat"] _] -> [_ _ _ _ w250]
                seq-local: [_ _ _ w240 _] -> [_ _ _ _ w249]
                tunnel: [w212 _ _ _ _] -> w196
                tunnel: [w211 _ _ _ _] -> w195
                tunnel: [dbl[] [6.7304, 0.0, 5.356, 5.9831, 0.0, 6.0646] ("ER 1-2") _ _ _ _] -> w194
                tunnel: [dbl[] [6.0887, 0.0, 4.9169, 5.2753, 0.0, 5.5338] ("ER 1-3") _ _ _ _] -> w193
                tunnel: [dbl[] [6.1683, 0.0, 5.0447, 5.2485, 0.0, 5.6703] ("ER 1-4") _ _ _ _] -> w192
                tunnel: [dbl[] [6.3872, 0.0, 5.0918, 5.4196, 0.0, 5.8365] ("ER 2-3") _ _ _ _] -> w191
                tunnel: [dbl[] [152.0, 22.0, 150.0, 147.0, 23.0, 151.0] ("T-A") _ _ _ _] -> w190
                tunnel: [dbl[] [149.0, 23.0, 153.0, 149.0, 23.0, 150.0] ("T-B") _ _ _ _] -> w189
                tunnel: [dbl[] [10058.0, 0.0, 5018.0, 4993.0, 0.0, 904.0] ("Pc") _ _ _ _] -> w188
                tunnel: [dbl[] [7492.0, 0.0, 3520.0, 3488.0, 0.0, 508.0] ("Pp") _ _ _ _] -> w187
                tunnel: [w213 _ _ _ _] -> w186
                tunnel: [timestamp[] [timestamp(3199615260.25 s since 1904-01-01), timestamp(3199586400.25 s since 1904-01-01), timestamp(3199635000.25 s since 1904-01-01), timestamp(3199623780.25 s since 1904-01-01), timestamp(3199586400.25 s since 1904-01-01), timestamp(3199669020.25 s since 1904-01-01)] ("Last Time") _ _ _ _] -> w185
                tunnel: [dbl[] [789.0, 0.0, 107.6, 105.8, 0.0, 51.2] ("Run Time") _ _ _ _] -> w184
                tunnel: [w200 _ _ _ _] -> w183
                tunnel: [dbl[] [1.234, 0.0, 3.456, 4.567, 0.0, 6.789] ("F 2-3") _ _ _ _] -> w182
                tunnel: [dbl[] [7492.0, 0.0, 3520.0, 3488.0, 0.0, 508.0] ("Pp") _ _ _ _] -> w181
                tunnel: [dbl[] [7492.0, 0.0, 3520.0, 3488.0, 0.0, 508.0] ("Pp") _ _ _ _] -> w180
                frame #0 {
                  w200 = dbl[] [123456789.0, 123456789.0, 123456789.0, 123456789.0, 123456789.0, 123456789.0]  # Next Time
                  w213 = dbl[] [12.345, 0.0, 2.509, 2.736, 0.0, 1.983] ("Pore Vol")
                  w211 = string[] ["Sample #1", "", "Sample #3", "Sample #4", "", "Sample #6"] ("Sample ID")
                  w212 = bool[] [TRUE, FALSE, TRUE, TRUE, FALSE, TRUE] ("Run")
                  # "Dummy Data"
                }
                frame #1 {
                  w214 = dbl[] [34.56, 0.0, 19.45, 25.04, 0.0, 71.38]  # Porosity
                  w215 = dbl[] [1.005, 0.0, 1.02, 0.996, 0.0, 2.034]  # Diameter
                  w217 = string[] ["Oil-Gas", "", "Water-Oil", "Water-Oil", "", "Gas-Water"]  # Fluid Pair
                  w216 = dbl[] [2.003, 0.0, 1.997, 2.017, 0.0, 4.056]  # Length
                  w218 = string[] ["Berea", "", "Sandstone", "Granite", "", "Shale"]  # Rock Type
                  w219 = string[] ["Project C1", "", "Project C3", "Project C4", "", "Project C6B"]  # Project
                  w224 = T3 [enum."Cell 1", enum."Cell 2", enum."Cell 3", enum."Cell 4", enum."Cell 5", enum."Cell 6B"] items=["Cell 1", "Cell 2", "Cell 3", "Cell 4", "Cell 5", "Cell 6A", "Cell 6B", "Cell 6C"]
                  n91 = for {
                    tunnel: w223 -> [w226] mode=indexing
                    tunnel: enum16{"Inactive", "Setup", "Active", "Done"}."Active" ("Cell Status") -> [w228]
                    tunnel: enum16{"Inactive", "Setup", "Active", "Done"}."Inactive" ("Cell Status") -> [w227]
                    tunnel: [w225] -> w220 mode=indexing
                    n92 = Select(t=w228, s=w226, f=w227) -> (s? t:f=w225:enum16{"Inactive", "Setup", "Active", "Done"})
                  }
                }
                frame #2 {
                  w230 = u32[] [3600, 0, 7200, 7200, 0, 10800]  # DAQ Period
                  w233 = dbl[] [1.1, 0.0, 1.3, 1.4, 0.0, 1.6]  # Amplitude
                  w234 = dbl[] [1000.0, 0.0, 3000.0, 4000.0, 0.0, 6000.0]  # Frequency
                  w235 = dbl[] [1.003, 0.0, 1.007, 0.999, 0.0, 2.031]  # Electrode Spacing
                  w236 = dbl[] [456.3, 0.0, 1056.2, 1234.5, 0.0, 5678.9]  # Permeability
                  n93 = Get Date/Time In Seconds() -> (seconds since 1Jan1904=w232:timestamp)
                  n94 = To Unsigned Long Integer(number=w232) -> (unsigned 32bit integer=w231:u32)
                  n95 = for {
                    tunnel: w231 -> [w239]
                    tunnel: w230 -> [w238] mode=indexing
                    tunnel: [w237] -> w229 mode=indexing
                    n96 = Add(x=w239, y=w238) -> (x+y=w237:u32)
                  }
                }
                frame #3 {
                  n97 = Initialize Array(0.0 ("element")) -> (w241:dbl[][])  [unwired: 2 in]
                  n98 = Build Array(w241, w241, w241, w241, w241, w241) -> (w240:dbl[][][])
                }
                frame #4 {
                  n99 = global read "Global ER2007.vi" "Test Info"() -> (w245:T4)
                  n100 = Unbundle By Name(w245) -> ("Cell Data"=w247:T5)
                  n101 = Index Array(array=w247) -> (element=w248:T6)  [unwired: 1 in]
                  n102 = for {
                    tunnel: w248 -> [w287]
                    tunnel: w267 -> [w286] mode=indexing
                    tunnel: [w285] -> w266 mode=indexing
                    tunnel: w265 -> [w284] mode=indexing
                    tunnel: w264 -> [w283] mode=indexing
                    tunnel: w263 -> [w282] mode=indexing
                    tunnel: w262 -> [w281] mode=indexing
                    tunnel: w261 -> [w280] mode=indexing
                    tunnel: w260 -> [w279] mode=indexing
                    tunnel: w259 -> [w278] mode=indexing
                    tunnel: w258 -> [w277] mode=indexing
                    tunnel: w257 -> [w276] mode=indexing
                    tunnel: w256 -> [w275] mode=indexing
                    tunnel: w255 -> [w274] mode=indexing
                    tunnel: w254 -> [w273] mode=indexing
                    tunnel: w253 -> [w272] mode=indexing
                    tunnel: w252 -> [w271] mode=indexing
                    tunnel: w251 -> [w270] mode=indexing
                    tunnel: w250 -> [w269] mode=indexing
                    tunnel: w249 -> [w268] mode=indexing
                    n103 = Bundle By Name(cluster=w287, "Cell ID"=w286, "Cell Status"=w284, "Project"=w282, "Sample #"=w283, "Rock Type"=w281, "Fluid Pair"=w280, "Length"=w279, "Diameter"=w278, "Porosity"=w277, "Permeability"=w276, "ElectSpace"=w275, "Frequency"=w274, "Amplitude"=w273, "DAQ Period"=w271, "Next Time"=w270, "Datafile"=w269, "Last Pore Vol"=w272, "CurData"=w268) -> (w285:T6)
                  }
                  n104 = Bundle By Name(cluster=w245, "CurCell"=0, "Cell Data"=w266) -> (w246:T4)
                  n105 = global write "Global ER2007.vi" "Test Info"(w246) -> ()
                }
              }
            }
            frame False {
              # "Read Cell Status file"
              n106 = stacked-sequence {
                seq-local: [w308 _ _] -> [_ w327 _]
                seq-local: [w310 _ _] -> [_ w328 _]
                seq-local: [w309 _ _] -> [_ _ w376]
                seq-local: [_ w326 _] -> [_ _ w375]
                tunnel: [w323 _ _] -> w304
                tunnel: [w322 _ _] -> w303
                tunnel: [w321 _ _] -> w302
                tunnel: [w320 _ _] -> w301
                tunnel: [w319 _ _] -> w300
                tunnel: [w317 _ _] -> w299
                tunnel: [w316 _ _] -> w298
                tunnel: [w315 _ _] -> w297
                tunnel: [w314 _ _] -> w296
                tunnel: [w313 _ _] -> w295
                tunnel: [_ w324 _] -> w294
                tunnel: [w311 _ _] -> w293
                tunnel: [w310 _ _] -> w292
                tunnel: [w312 _ _] -> w291
                tunnel: [w318 _ _] -> w290
                tunnel: [w306 _ _] -> w289
                tunnel: [w305 _ _] -> w288
                frame #0 {
                  # "Reads the actual Cell Status file"
                  n107 = global read "Global ER2007.vi" "Status File Path"() -> (w307:path)
                  n108 = call "Read Cell Status File.vi"("FilePathIn"=w307) -> ("Pdn"=w305:dbl[], "Pdp"=w306:dbl[], "Next Time"=w312:dbl[], "Run Status"=w310:bool[], "Elapsed-T"=w311:dbl[], "SampID"=w323:string[], "ER 1-2"=w322:dbl[], "Pv"=w313:dbl[], "ER 1-3"=w321:dbl[], "Pp"=w314:dbl[], "ER 1-4"=w320:dbl[], "Pc"=w315:dbl[], "Test Info"=w309:T4, "ER 2-3"=w319:dbl[], "F 2-3"=w318:dbl[], "TA"=w317:dbl[], "TB"=w316:dbl[])  [unwired: 4 in, 6 out]
                  n109 = Unbundle By Name(w309) -> ("Cell Data"=w308:T5)
                }
                frame #1 {
                  w325 = TRUE  # Rd All ?
                  # "Get existing data and last time"
                  n110 = for {
                    tunnel: w327 -> [w337] mode=indexing
                    tunnel: w328 -> [_] mode=indexing
                    shift-right: [w341] -> w326
                    shift-left: w327 -> [w342]
                    tunnel: [w339] -> w324 mode=indexing
                    tunnel: w325 -> [w331]
                    i -> [w340]
                    n111 = Unbundle By Name(w337) -> ("Start Time"=w330:dbl, "Datafile"=w335:path)
                    n112 = Path To String(path=w335) -> (string=w334:string)
                    n113 = Not Equal To 0?(x=w330) -> (x != 0?=w336:bool)
                    n114 = String Length(string=w334) -> (length=w333:i32)
                    n115 = Greater?(x=w333, y=5) -> (0:w329:bool)
                    n116 = Compound Arithmetic op=AND(w331, w336, w329) -> (w338:bool)
                    n117 = case shown="True" w338 {
                      tunnel: w342 -> [w344 w362]
                      tunnel: [w344 w361] -> w341
                      tunnel: w337 -> [_ w359]
                      tunnel: w340 -> [_ w358]
                      tunnel: [timestamp(0 s since 1904-01-01) ("*(type *) &x") w347] -> w339
                      tunnel: w335 -> [_ w346]
                      tunnel: w330 -> [_ w345]
                      frame False {
                        # "This cell wasn't active"
                      }
                      frame True {
                        w352 = sgl 3600.0  # To secs
                        w364 = TRUE  # ErrMsgOff
                        # "gets last elapsed time in hrs, adds to\nStart Time to get last clock time"
                        # "Reads the cell's data file"
                        n118 = Strip Path(path=w346) -> (stripped path=w366:path, name=w365:string)
                        n119 = call "Read Header and Spreadsheet File.vi"("DirIn"=w366, "NameIn"=w365, "ErrMsgOff"=w364) -> ("2D Data"=w354:sgl[][], "Error Out"=w363:errorcluster)  [unwired: 10 in, 5 out]
                        n120 = Unbundle By Name(w363) -> ("status"=w360:bool)
                        n121 = case shown="False" w360 {
                          tunnel: w362 -> [w372 w373]
                          tunnel: [w371 w373] -> w361
                          tunnel: w359 -> [w370 _]
                          tunnel: w354 -> [w369 _]
                          tunnel: w358 -> [w368 _]
                          frame False {
                            n122 = Bundle By Name(cluster=w370, "CurData"=w369) -> (w367:T6)
                            n123 = Replace Array Subset(array=w372, new element=w367, index=w368) -> (w371:T5)
                          }
                          frame True {
                            # "Error"
                          }
                        }
                        n124 = Index Array(array=w354, index (col)=0 ("disabled index (col)")) -> (element=w356:sgl[])  [unwired: 1 in]
                        n125 = Array Size(array=w356) -> (size(s)=w355:i32)
                        n126 = Decrement(x=w355) -> (x-1=w350:i32)
                        n127 = Index Array(array=w354, index (row)=w350, index (col)=0 ("index (row)")) -> (element=w353:sgl)
                        n128 = Multiply(x=w352, y=w353) -> (x*y=w351:sgl)
                        n129 = Add(x=w351, y=w345) -> (x+y=w348:dbl)
                        n130 = To Time Stamp(1:w348) -> (0:w347:timestamp)
                      }
                    }
                  }
                }
                frame #2 {
                  # "Final values"
                  n131 = Bundle By Name(cluster=w376, "Cell Data"=w375) -> (w374:T4)
                  n132 = global write "Global ER2007.vi" "Test Info"(w374) -> ()
                }
              }
            }
          }
          n133 = local write item#-1("Radio Cell Selects") -> ()
          n134 = case shown="\"CS 1\", Default" "Radio Cell Selects" {
            tunnel: [u8 2 ("Disabled") u8 0 ("Disabled")] -> w179
            frame "No Selection" {
            }
            frame "CS 1", Default {
            }
          }
          n135 = property on="TakePt" class="Bool"("Disabled"=w179) -> ()  [unwired: 2 in, 2 out]
          n136 = property on="Setup" class="Bool"("Disabled"=w179) -> ()  [unwired: 2 in, 2 out]
          n137 = property on="History" class="Bool"("Disabled"=w179) -> ()  [unwired: 2 in, 2 out]
          n138 = local write "ER 1-2"(w175) -> ()
          n139 = local write "ER 2-3"(w172) -> ()
          n140 = local write "ER 1-3"(w174) -> ()
          n141 = local write "ER 1-4"(w173) -> ()
          n142 = local write "F 2-3"(w163) -> ()
          n143 = local write item#-1(w166) -> ()
          n144 = local write item#-1(w171) -> ()
          n145 = local write item#-1(w170) -> ()
          n146 = local write item#-1(w168) -> ()
          n147 = local write item#-1(w160) -> ()
          n148 = local write item#-1(w176) -> ()
          n149 = local write item#-1(w169) -> ()
          n150 = local write item#-1(w161) -> ()
          n151 = local write item#-1(w165) -> ()
          n152 = local write item#-1(w167) -> ()
        }
        frame #8 {
          w381 = TRUE  # Init
          # "Other PC Idx"
          # "Inits the Sample Request vi"
          n153 = call "Sample Request Control.vi"("PC ID"=w380, "SimOn"=w383, "Init"=w381) -> ("ErrOut"=w382:errorcluster)  [unwired: 11 in, 5 out]
          n154 = case shown="1, Default" w380 {
            tunnel: [1 ("index") 0 ("index")] -> w379
            frame 1, Default {
            }
            frame 2 {
            }
          }
          n155 = call <vilib>:"Simple Error Handler.vi"("error in (no error)"=w382) -> ()  [unwired: 4 in, 5 out]
        }
        frame #9 {
          # "Starts the Background DAQ Task running"
          n156 = global read "Global ER2007.vi" "BckDaqLp vi name"() -> (w387:path)
          n157 = Array Size(array=w391) -> (size(s)=w390:i32)
          n158 = global read "Global ER2007.vi" "DAQ Run"() -> (w386:bool)
          n159 = Initialize Array(FALSE, w390) -> (w388:bool[])
          n160 = case shown="False" w386 {
            tunnel: w387 -> [w392 w399]
            frame False {
              # "Not running - start it up"
              n161 = stacked-sequence {
                tunnel: w392 -> [_ w394]
                frame #0 {
                  # "Set the Init flag"
                  n162 = global write "Global ER2007.vi" "DAQ Init"(TRUE ("A/D Init")) -> ()
                }
                frame #1 {
                  # "Run it"
                  n163 = Open VI Reference(vi path=w394) -> (vi reference=w398:refnum<vi>)  [unwired: 5 in, 1 out]
                  n164 = invoke class="VI" method="Run VI"(reference=w398, "Wait until done"=FALSE, "Auto Dispose Ref"=TRUE) -> (error out=w395:errorcluster)  [unwired: 2 in, 4 out]
                  n165 = call <vilib>:"Simple Error Handler.vi"("error in (no error)"=w395) -> ()  [unwired: 4 in, 5 out]
                }
              }
            }
            frame True {
              # "The bckgnd task is already running - stop it and restart"
              n166 = stacked-sequence {
                tunnel: w399 -> [_ _ _ w403]
                frame #0 {
                  # "Stop the task"
                  n167 = global write "Global ER2007.vi" "DAQ Stop"(TRUE ("A/D Stop")) -> ()
                }
                frame #1 {
                  # "Small wait"
                  n168 = Wait (ms)(milliseconds to wait=u32 500) -> ()  [unwired: 1 out]
                }
                frame #2 {
                  # "Set the Init flag"
                  n169 = global write "Global ER2007.vi" "DAQ Init"(TRUE ("A/D Init")) -> ()
                }
                frame #3 {
                  # "Restart the task"
                  n170 = Open VI Reference(vi path=w403) -> (vi reference=w407:refnum<vi>)  [unwired: 5 in, 1 out]
                  n171 = invoke class="VI" method="Run VI"(reference=w407, "Wait until done"=FALSE, "Auto Dispose Ref"=TRUE) -> (error out=w404:errorcluster)  [unwired: 2 in, 4 out]
                  n172 = call <vilib>:"Simple Error Handler.vi"("error in (no error)"=w404) -> ()  [unwired: 4 in, 5 out]
                }
              }
            }
          }
        }
        frame #10 {
          # "Starts the Get Cell Data background task"
          n173 = global read "Global ER2007.vi" "BckGetEng vi name"() -> (w408:path)
          n174 = stacked-sequence {
            tunnel: w408 -> [_ _ w412]
            frame #0 {
              w409 = FALSE ("GCD Go")
              # "Clears flags"
              n175 = global write "Global ER2007.vi" "GCD Go"(w409) -> ()
              n176 = global write "Global ER2007.vi" "GCD Err"(w409) -> ()
              n177 = global write "Global ER2007.vi" "GCD Busy"(w409) -> ()
              n178 = global write "Global ER2007.vi" "GCD Stop"(w409) -> ()
            }
            frame #1 {
              # "Small wait"
              n179 = Wait (ms)(milliseconds to wait=u32 500) -> ()  [unwired: 1 out]
            }
            frame #2 {
              # "If task is running, stop it; otherwise just start it"
              n180 = global read "Global ER2007.vi" "GCD Run"() -> (w411:bool)
              n181 = case shown="True" w411 {
                tunnel: w412 -> [w413 w419]
                frame False {
                  n182 = stacked-sequence {
                    tunnel: w413 -> [w414]
                    frame #0 {
                      n183 = Open VI Reference(vi path=w414) -> (vi reference=w415:refnum<vi>)  [unwired: 5 in, 1 out]
                      n184 = invoke class="VI" method="Run VI"(reference=w415, "Wait until done"=FALSE, "Auto Dispose Ref"=TRUE) -> (error out=w418:errorcluster)  [unwired: 2 in, 4 out]
                      n185 = call <vilib>:"Simple Error Handler.vi"("error in (no error)"=w418) -> ()  [unwired: 4 in, 5 out]
                    }
                  }
                }
                frame True {
                  # "task is still running"
                  n186 = stacked-sequence {
                    tunnel: w419 -> [_ _ _ _ w435]
                    frame #0 {
                      # "stops task"
                      n187 = global write "Global ER2007.vi" "GCD Stop"(TRUE ("GCD Stop")) -> ()
                    }
                    frame #1 {
                      # "Small wait"
                      n188 = Wait (ms)(milliseconds to wait=u32 500) -> ()  [unwired: 1 out]
                    }
                    frame #2 {
                      # "Waits for task to stop or timeout"
                      n189 = Get Date/Time In Seconds() -> (seconds since 1Jan1904=w423:timestamp)
                      n190 = To Double Precision Float(number=w423) -> (double precision float=w422:dbl)
                      n191 = while {
                        tunnel: w422 -> [w431]
                        stop <- w426 stop-if-true
                        n192 = Get Date/Time In Seconds() -> (seconds since 1Jan1904=w433:timestamp)
                        n193 = global read "Global ER2007.vi" "GCD Stop"() -> (w424:bool)
                        n194 = To Double Precision Float(number=w433) -> (double precision float=w432:dbl)
                        n195 = Wait Until Next ms Multiple(millisecond multiple=u32 250) -> ()  [unwired: 1 out]
                        n196 = Subtract(x=w432, y=w431) -> (x-y=w430:dbl)
                        n197 = Greater?(x=w430, y=8.0) -> (0:w427:bool)
                        n198 = Not(x=w424) -> (.not. x?=w425:bool)
                        n199 = Or(x=w427, y=w425) -> (x .or. y?=w426:bool)
                      }
                    }
                    frame #3 {
                      # "Small wait"
                      n200 = Wait (ms)(milliseconds to wait=u32 500) -> ()  [unwired: 1 out]
                    }
                    frame #4 {
                      # "Run it"
                      n201 = Open VI Reference(vi path=w435) -> (vi reference=w439:refnum<vi>)  [unwired: 5 in, 1 out]
                      n202 = invoke class="VI" method="Run VI"(reference=w439, "Wait until done"=FALSE, "Auto Dispose Ref"=TRUE) -> (error out=w436:errorcluster)  [unwired: 2 in, 4 out]
                      n203 = call <vilib>:"Simple Error Handler.vi"("error in (no error)"=w436) -> ()  [unwired: 4 in, 5 out]
                    }
                  }
                }
              }
            }
          }
        }
      }
    }
    frame #1 {
      # "Main\nloop"
      n204 = while {
        shift-right: [w475] -> _
        shift-left: w451 -> [w468]
        shift-right: [w476] -> _
        shift-left: w450 -> [w477]
        shift-right: [FALSE ("Init")] -> _
        shift-left: w449 -> [w474]
        shift-right: [w472] -> _
        shift-left: w448 -> [w471]
        shift-right: [w469] -> _
        shift-left: w447 -> [w470]
        shift-right: [w465] -> _
        shift-left: w445 -> [w466]
        shift-right: [w467] -> _
        shift-left: w446 -> [w464]
        shift-right: [w463] -> _
        shift-left: w444 -> [w462]
        shift-right: [w460] -> _
        shift-left: w443 -> [w461]
        tunnel: w442 -> [w455]
        tunnel: w441 -> [w454]
        shift-right: [w453] -> _
        shift-left: w440 -> [w452]
        stop <- w478 stop-if-true
        # "Stop IP"
        # "Refresh"
        # "Other PC Idx"
        # "Init"
        # "SimDAQ"
        # "CurSUPCell"
        # "CurGCDCell"
        # "CurSelectedCell"
        # "RadioSelect"
        # "TakePtActive"
        # "CurActiveCells"
        n205 = global read "Global ER2007.vi" "New Data"() -> (w459:bool)
        n206 = global read "Global ER2007.vi" "New Setup"() -> (w458:bool)
        n207 = global read "Global ER2007.vi" "GCD Prog"() -> (→"GCD Prog":bool[])
        n208 = global read "Global ER2007.vi" "TakePt"() -> (w457:bool)
        n209 = Wait Until Next ms Multiple(millisecond multiple=u32 333) -> ()  [unwired: 1 out]
        n210 = event shown="[0] Timeout" {
          selector: _ -> [_ _ _ _ _ _ _ _ _]
          dyn-events: _ -> [_ _ _ _ _ _ _ _ _]
          timeout: 333 -> [_ _ _ _ _ _ _ _ _]
          tunnel: [w499 w1163 w1182 w1209 w1237 w1272 w1283 w1302 w1313] -> w475
          tunnel: w468 -> [w500 w1163 w1182 w1209 w1237 w1272 w1283 w1302 w1313]
          tunnel: [w483 FALSE FALSE FALSE FALSE FALSE FALSE FALSE FALSE] -> w478
          tunnel: w477 -> [w487 _ w1181 w1208 w1236 w1273 w1282 w1303 w1314]
          tunnel: [w487 w1161 w1181 w1208 w1236 w1273 w1282 w1303 w1314] -> w476
          tunnel: w457 -> [w502 _ _ _ _ _ _ _ _]
          tunnel: w458 -> [w505 _ _ _ _ _ _ _ _]
          tunnel: w459 -> [w503 _ _ _ _ _ _ _ _]
          tunnel: w474 -> [w501 _ _ _ _ _ _ _ _]
          tunnel: [w498 w1162 w1180 w1207 w1235 w1262 w1281 w1301 w1312] -> w472
          tunnel: w471 -> [w497 w1162 w1180 w1207 w1235 w1262 w1281 w1301 w1312]
          tunnel: w470 -> [w485 w1160 w1179 w1206 w1234 w1261 w1280 w1300 w1311]
          tunnel: [w496 w1160 w1179 w1206 w1234 w1261 w1280 w1300 w1311] -> w469
          tunnel: w464 -> [w493 w1159 w1178 w1205 w1233 w1259 w1278 w1297 w1309]
          tunnel: [w494 w1159 w1178 w1205 w1233 w1259 w1278 w1297 w1309] -> w467
          tunnel: w466 -> [w492 w1158 w1177 w1203 w1232 w1260 w1279 w1299 w1310]
          tunnel: [w495 w1157 w1177 w1203 w1232 w1260 w1279 w1299 w1310] -> w465
          tunnel: [w490 w1156 w1176 w1204 w1231 w1258 w1277 w1298 w1308] -> w463
          tunnel: w462 -> [w491 w1156 w1176 _ w1231 w1258 w1277 w1298 w1308]
          tunnel: w461 -> [w489 _ w1175 w1202 w1230 w1257 w1276 w1296 w1307]
          tunnel: [w488 TRUE w1175 w1202 w1230 w1257 w1276 w1296 w1307] -> w460
          tunnel: w455 -> [w486 _ _ _ _ _ _ _ _]
          tunnel: w454 -> [w484 _ _ _ _ _ _ _ _]
          tunnel: [w481 w1154 w1174 w1201 w1229 w1256 w1275 w1294 TRUE] -> w453
          tunnel: w452 -> [w482 w1154 w1174 w1201 w1229 w1256 w1275 w1294 _]
          event Timeout {
            # "Timeout"
            n211 = event-data() -> ()  [unwired: 1 in, 1 out]
            n212 = Compound Arithmetic op=OR(w503, w505, w502, w501) -> (w504:bool)
            n213 = case shown="False" w504 {
              tunnel: w503 -> [_ w819]
              tunnel: w502 -> [_ w818]
              tunnel: w500 -> [w522 w807]
              tunnel: [w521 w806] -> w499
              tunnel: [w523 w811] -> w498
              tunnel: w497 -> [w523 w810]
              tunnel: w485 -> [w520 w809]
              tunnel: [w519 w808] -> w496
              tunnel: w492 -> [w518 w802]
              tunnel: [w517 w802] -> w495
              tunnel: [w516 w805] -> w494
              tunnel: w493 -> [w515 w805]
              tunnel: w491 -> [w514 w803]
              tunnel: [w513 w804] -> w490
              tunnel: w489 -> [w512 _]
              tunnel: [w511 w801] -> w488
              tunnel: w486 -> [w510 _]
              tunnel: w484 -> [w509 _]
              tunnel: [w508 FALSE] -> w483
              tunnel: w482 -> [w507 w796]
              tunnel: [w506 w796] -> w481
              frame False {
                n214 = stacked-sequence {
                  seq-local: [w535 _ _] -> [_ w622 _]
                  seq-local: [w530 _ _] -> [_ w621 _]
                  seq-local: [w546 _ _] -> [_ w618 _]
                  seq-local: [w542 _ _] -> [_ w613 _]
                  tunnel: w523 -> [w552 _ _]
                  tunnel: w522 -> [w551 w620 _]
                  tunnel: [_ w619 _] -> w521
                  tunnel: w520 -> [w550 w611 _]
                  tunnel: [_ w612 _] -> w519
                  tunnel: w518 -> [_ w615 w751]
                  tunnel: [_ _ w751] -> w517
                  tunnel: [_ w617 _] -> w516
                  tunnel: w515 -> [w547 w614 _]
                  tunnel: w514 -> [w545 _ w750]
                  tunnel: [_ _ w749] -> w513
                  tunnel: w512 -> [w541 _ _]
                  tunnel: [_ w616 _] -> w511
                  tunnel: w510 -> [w532 _ _]
                  tunnel: w509 -> [w529 _ _]
                  tunnel: [_ _ w743] -> w508
                  tunnel: w507 -> [_ _ w745]
                  tunnel: [_ _ w744] -> w506
                  frame #0 {
                    # "TRUE if time to sample a cell"
                    # "Sample cell index"
                    # "Checks if sample req'd"
                    n215 = local read "GCD Busy"() -> (w543:bool)
                    n216 = global read "Global ER2007.vi" "GCD Busy"() -> (w538:bool)
                    n217 = Get Date/Time In Seconds() -> (seconds since 1Jan1904=w549:timestamp)
                    n218 = global read "Global ER2007.vi" "GCD Err"() -> (→"GCD Err":bool)
                    n219 = To Double Precision Float(number=w549) -> (double precision float=w548:dbl)
                    "Cur Time" <- w548
                    n220 = Not Equal?(x=w543, y=w538) -> (x != y?=w544:bool)
                    n221 = case shown="True" w538 {
                      tunnel: w552 -> [w565 _]
                      tunnel: w551 -> [w575 _]
                      tunnel: [w574 0] -> w530
                      tunnel: [w573 w609] -> w534
                      tunnel: w550 -> [w572 _]
                      tunnel: w548 -> [w570 _]
                      tunnel: w545 -> [w568 _]
                      frame False {
                        n222 = case shown="0, Default" w568 {
                          tunnel: [-1 0 1 2 3 4] -> w569
                          frame 0, Default {
                          }
                          frame 1 {
                          }
                          frame 2 {
                          }
                          frame 3 {
                          }
                          frame 4 {
                          }
                          frame 5 {
                          }
                        }
                        n223 = Array Size(array=w565) -> (size(s)=w567:i32)
                        n224 = Or Array Elements(Boolean array=w572) -> (logical OR=w571:bool)
                        n225 = Decrement(x=w567) -> (x-1=w566:i32)
                        n226 = case shown="True" w571 {
                          tunnel: w565 -> [w588 _]
                          tunnel: w575 -> [w587 _]
                          tunnel: [w586 w604] -> w574
                          tunnel: [w585 w605] -> w573
                          tunnel: w572 -> [_ w606]
                          tunnel: w570 -> [w584 _]
                          tunnel: w569 -> [w583 _]
                          tunnel: w566 -> [w582 _]
                          frame False {
                            # "Normal sample checker"
                            n227 = while {
                              tunnel: w588 -> [w599] mode=indexing
                              tunnel: w582 -> [w598]
                              tunnel: w587 -> [w597] mode=indexing
                              tunnel: w584 -> [w596]
                              tunnel: [w592] -> w586
                              tunnel: [w595] -> w585
                              tunnel: w583 -> [w593]
                              i -> [w592]
                              stop <- w591 stop-if-true
                              # "NOT current SUP cell"
                              n228 = case shown="True" w599 {
                                tunnel: w597 -> [_ w602]
                                tunnel: w596 -> [_ w603]
                                tunnel: [FALSE w601] -> w595
                                frame False {
                                # "Not Active"
                                }
                                frame True {
                                # "This cell is active - see\nif is time for a sample"
                                n229 = Less Or Equal?(x=w602, y=w603) -> (x <= y?=w601:bool)
                                }
                              }
                              n230 = Not Equal?(x=w592, y=w593) -> (x != y?=w589:bool)
                              n231 = Less Or Equal?(x=w598, y=w592) -> (x <= y?=w594:bool)
                              n232 = Or(x=w595, y=w594) -> (x .or. y?=w590:bool)
                              n233 = And(x=w590, y=w589) -> (x .and. y?=w591:bool)
                            }
                          }
                          frame True {
                            w605 = TRUE  # Take Pt Sample
                            # "TakePt is active"
                            n234 = while {
                              tunnel: w606 -> [w607] mode=indexing
                              tunnel: [w608] -> w604
                              i -> [w608]
                              stop <- w607 stop-if-true
                            }
                          }
                        }
                      }
                      frame True {
                        w609 = FALSE  # Don't sample
                        # "\"Get Cell Data.vi\" is still busy"
                      }
                    }
                    n235 = case shown="True" w544 {
                      tunnel: w547 -> [w558 w562]
                      tunnel: [w558 w561] -> w546
                      tunnel: w538 -> [_ w560]
                      tunnel: [w557 TRUE] -> w542
                      tunnel: w541 -> [w557 _]
                      frame False {
                      }
                      frame True {
                        n236 = case shown="False" w560 {
                          tunnel: w562 -> [_ w564]
                          tunnel: [w563 w564] -> w561
                          frame False {
                            w563 = 0  # <none>
                          }
                          frame True {
                          }
                        }
                        "GCD Busy" <- w560
                      }
                    }
                    n237 = global read "Global ER2007.vi" "DAQ Run"() -> (→"DAQ Run":bool)
                    n238 = local read "System Error"() -> (w539:bool)
                    n239 = global read "Global ER2007.vi" "A/D Err"() -> (w525:bool)
                    n240 = global read "Global ER2007.vi" "Galil Err"() -> (w526:bool)
                    n241 = Or(x=w525, y=w526) -> (x .or. y?=w524:bool)
                    n242 = Not Equal?(x=w539, y=w524) -> (x != y?=w540:bool)
                    n243 = case shown="True" w540 {
                      tunnel: w524 -> [_ w554]
                      tunnel: w526 -> [_ w555]
                      tunnel: w525 -> [_ w556]
                      frame False {
                      }
                      frame True {
                        n244 = property on="System Error" class="Bool (strict)"("Visible"=w554) -> ()  [unwired: 2 in, 2 out]
                        n245 = property on="Reset DAQ" class="Bool"("Visible"=w554) -> ()  [unwired: 2 in, 2 out]
                        "A/D Err" <- w556
                        "System Error" <- w554
                        "VPA Err" <- w555
                      }
                    }
                    n246 = global read "Global ER2007.vi" "GCD Reset"() -> (w531:bool)
                    "GCD Reset" <- w531
                    n247 = call "Sample Request Control.vi"("Sample Request"=w534, "SimOn"=w532, "Reset"=w531) -> ("Request Granted"=w535:bool, "Reset Done"=w533:bool, "Busy Status"=w527:bool[])  [unwired: 11 in, 3 out]
                    n248 = case shown="True" w533 {
                      frame False {
                      }
                      frame True {
                        n249 = global write "Global ER2007.vi" "GCD Reset"(FALSE ("GCD Reset")) -> ()
                      }
                    }
                    n250 = Index Array(array=w527, index=w529) -> (element=→"Other PC Busy":bool)
                    n251 = global write "Global ER2007.vi" "BoxBusy"(w527) -> ()
                  }
                  frame #1 {
                    n252 = case shown="True" w622 {
                      tunnel: w621 -> [_ w680]
                      tunnel: w620 -> [w628 w679]
                      tunnel: [w628 w678] -> w619
                      tunnel: [w625 w677] -> w617
                      tunnel: w618 -> [w625 _]
                      tunnel: [w627 TRUE] -> w616
                      tunnel: w615 -> [w626 _]
                      tunnel: w614 -> [_ _]
                      tunnel: w613 -> [w624 _]
                      tunnel: [w623 w675] -> w612
                      tunnel: w611 -> [w623 w674]
                      frame False {
                        # "No sample req'd or possible at this time"
                        n253 = case shown="True" w624 {
                          tunnel: [FALSE FALSE] -> w627
                          tunnel: w626 -> [_ w636]
                          tunnel: w625 -> [_ w631]
                          tunnel: w623 -> [_ w630]
                          frame False {
                          }
                          frame True {
                            # "Update control visible properties"
                            n254 = case shown="1, Default" w636 {
                              selector: w636 -> [_ w648]
                              tunnel: [u8 2 ("Disabled") w650] -> w635
                              tunnel: [u8 2 ("Disabled") w642] -> w634
                              tunnel: [u8 2 ("Disabled") w655] -> w633
                              tunnel: [u8 0 ("Disabled") u8 0 ("Disabled")] -> w632
                              tunnel: w631 -> [_ w652]
                              tunnel: w630 -> [_ w646]
                              frame 0 {
                              }
                              frame 1, Default {
                                w643 = u8 2 ("Disabled")
                                # "TRUE if Radio button = CurGCDCell"
                                n255 = global read "Global ER2007.vi" "Test Info"() -> (w649:T4)
                                n256 = Or Array Elements(Boolean array=w646) -> (logical OR=w645:bool)
                                n257 = Decrement(x=w648) -> (x-1=w647:i32)
                                n258 = Equal?(x=w648, y=w652) -> (x = y?=w651:bool)
                                n259 = Unbundle By Name(w649) -> ("Cell Data"=w653:T5)
                                n260 = Index Array(array=w653, index=w647) -> (element=w673:T6)
                                n261 = Unbundle By Name(w673) -> ("Length"=w672:dbl, "Diameter"=w670:dbl, "ElectSpace"=w671:dbl, "CurData"=w663:dbl[][])
                                n262 = Less Or Equal To 0?(x=w671) -> (x <= 0?=w667:bool)
                                n263 = Less Or Equal To 0?(x=w672) -> (x <= 0?=w669:bool)
                                n264 = Index Array(array=w663, index (col)=0 ("disabled index (col)")) -> (element=w662:dbl[])  [unwired: 1 in]
                                n265 = Less Or Equal To 0?(x=w670) -> (x <= 0?=w668:bool)
                                n266 = Array Size(array=w662) -> (size(s)=w661:i32)
                                n267 = Select(t=u8 2 ("Disabled"), s=w651, f=u8 0) -> (s? t:f=w650:u8)
                                n268 = Compound Arithmetic op=OR(w669, w668, w667) -> (w666:bool)
                                n269 = Less?(x=w661, y=2) -> (x < y?=w660:bool)
                                n270 = Select(t=w643, s=w666, f=w650) -> (s? t:f=w644:u8)
                                n271 = Select(t=u8 2 ("Disabled"), s=w660, f=u8 0 ("Disabled")) -> (s? t:f=w655:u8)
                                n272 = Select(t=w643, s=w645, f=w644) -> (s? t:f=w642:u8)
                              }
                            }
                            n273 = property on="Setup" class="Bool"("Disabled"=w635) -> ()  [unwired: 2 in, 2 out]
                            n274 = property on="TakePt" class="Bool"("Disabled"=w634) -> ()  [unwired: 2 in, 2 out]
                            n275 = property on="History" class="Bool"("Disabled"=w633) -> ()  [unwired: 2 in, 2 out]
                            n276 = property on="CurVals" class="Bool"("Disabled"=w632) -> ()  [unwired: 2 in, 2 out]
                          }
                        }
                      }
                      frame True {
                        # "Sample\nreq'd"
                        n277 = stacked-sequence {
                          tunnel: w680 -> [w683 w707]
                          tunnel: w679 -> [w695 _]
                          tunnel: [w694 _] -> w678
                          tunnel: [w687 _] -> w677
                          tunnel: [w686 _] -> w675
                          tunnel: w674 -> [w685 _]
                          frame #0 {
                            # "Updates Next\nTime, sets flags"
                            n278 = global read "Global ER2007.vi" "Test Info"() -> (w690:T4)
                            n279 = Boolean To (0,1)(Boolean=w685) -> (0, 1=w684:i16[])
                            n280 = Unbundle By Name(w690) -> ("Cell Data"=w698:T5)
                            n281 = Index Array(array=w684, index=w683) -> (element=w682:i16)
                            n282 = Index Array(array=w698, index=w683) -> (element=w699:T6)
                            n283 = Greater Than 0?(x=w682) -> (x > 0?=w681:bool)
                            n284 = global write "Global ER2007.vi" "GCD Busy"(TRUE ("GCD Busy")) -> ()
                            n285 = Unbundle By Name(w699) -> ("Cell ID"=w687:i32, "DAQ Period"=w701:u32, "DAQ Units"=w700:u16, "Start Time"=w692:dbl, "Next Time"=w693:dbl)
                            "Selected Data Cell" <- w687
                            n286 = case shown="True" w681 {
                              tunnel: [w702 w704] -> w686
                              tunnel: w685 -> [w702 w703]
                              frame False {
                              }
                              frame True {
                                n287 = Array Size(array=w703) -> (size(s)=w706:i32)
                                n288 = Initialize Array(FALSE, w706) -> (w704:bool[])
                              }
                            }
                            n289 = call "Sample Timer Functions.vi"("Next Time In"=w693, "Start Time"=w692, "DAQ Units"=w700, "DAQ Period"=w701) -> ("New Time Out"=w691:dbl)  [unwired: 2 in, 5 out]
                            n290 = Replace Array Subset(array=w695, new element=w691, index=w683) -> (w694:dbl[])
                            n291 = Bundle By Name(cluster=w699, "Next Time"=w691) -> (w696:T6)
                            n292 = Replace Array Subset(array=w698, new element=w696, index=w683) -> (w697:T5)
                            n293 = Bundle By Name(cluster=w690, "CurCell"=w687, "Cell Data"=w697) -> (w689:T4)
                            n294 = global write "Global ER2007.vi" "Test Info"(w689) -> ()
                            n295 = global write "Global ER2007.vi" "DataCell"(w687) -> ()
                            "Cell Data Idx" <- w683
                          }
                          frame #1 {
                            w710 = cluster{u32, u32}[] [{1985280, 1985280}, {6618880, 6618880}, {1985280, 1985280}, {6618880, 6618880}]  # Busy Colors
                            # "Runs the \"Get Cell Data.vi\"; lights the\n\"Busy\" LED"
                            n296 = global read "Global ER2007.vi" "GCD Run"() -> (w708:bool)
                            n297 = case shown="False" w708 {
                              frame False {
                                # "NOT running for some reason"
                                n298 = stacked-sequence {
                                seq-local: [w712 _ _] -> [_ w719 _]
                                seq-local: [_ w718 _] -> [_ _ w729]
                                frame #0 {
                                n299 = global read "Global ER2007.vi" "BckGetEng vi name"() -> (w711:path)
                                n300 = Get Date/Time In Seconds() -> (seconds since 1Jan1904=w713:timestamp)
                                n301 = To Double Precision Float(number=w713) -> (double precision float=w712:dbl)
                                n302 = Open VI Reference(vi path=w711) -> (vi reference=w714:refnum<vi>)  [unwired: 5 in, 1 out]
                                n303 = invoke class="VI" method="Run VI"(reference=w714, "Wait until done"=FALSE, "Auto Dispose Ref"=TRUE) -> (error out=w717:errorcluster)  [unwired: 2 in, 4 out]
                                n304 = call <vilib>:"Simple Error Handler.vi"("error in (no error)"=w717) -> ()  [unwired: 4 in, 5 out]
                                }
                                frame #1 {
                                n305 = while {
                                tunnel: w719 -> [w726]
                                tunnel: [w721] -> w718
                                stop <- w722 stop-if-true
                                # "Waits for Run flag or T/O"
                                n306 = Get Date/Time In Seconds() -> (seconds since 1Jan1904=w728:timestamp)
                                n307 = To Double Precision Float(number=w728) -> (double precision float=w727:dbl)
                                n308 = global read "Global ER2007.vi" "GCD Run"() -> (w720:bool)
                                n309 = Wait Until Next ms Multiple(millisecond multiple=u32 250) -> ()  [unwired: 1 out]
                                n310 = Subtract(x=w727, y=w726) -> (x-y=w725:dbl)
                                n311 = Greater?(x=w725, y=2.0) -> (0:w721:bool)
                                n312 = Or(x=w721, y=w720) -> (x .or. y?=w722:bool)
                                }
                                }
                                frame #2 {
                                n313 = case shown="False" w729 {
                                frame False {
                                # "Get cell data"
                                n314 = global write "Global ER2007.vi" "GCD Go"(TRUE ("GCD Run")) -> ()
                                }
                                frame True {
                                # "T/O error"
                                n315 = global write "Global ER2007.vi" "GCD Busy"(FALSE ("GCD Busy")) -> ()
                                }
                                }
                                }
                                }
                              }
                              frame True {
                                # "Get cell data"
                                n316 = global write "Global ER2007.vi" "GCD Go"(TRUE ("GCD Run")) -> ()
                              }
                            }
                            n317 = case shown="1" w707 {
                              tunnel: w710 -> [w734 w735 w737 w739 w741]
                              tunnel: TRUE ("C1-Status") -> [w733 w736 w738 w740 w742]
                              frame 0, Default {
                                n318 = property on="C1-Status" class="Bool (strict)"("Value"=w733, "Colors [4]"=w734) -> ()  [unwired: 2 in, 2 out]
                              }
                              frame 1 {
                                n319 = property on="C2-Status" class="Bool (strict)"("Value"=w736, "Colors [4]"=w735) -> ()  [unwired: 2 in, 2 out]
                              }
                              frame 2 {
                                n320 = property on="C3-Status" class="Bool (strict)"("Value"=w738, "Colors [4]"=w737) -> ()  [unwired: 2 in, 2 out]
                              }
                              frame 3 {
                                n321 = property on="C4-Status" class="Bool (strict)"("Value"=w740, "Colors [4]"=w739) -> ()  [unwired: 2 in, 2 out]
                              }
                              frame 4 {
                                n322 = property on="C5-Status" class="Bool (strict)"("Value"=w742, "Colors [4]"=w741) -> ()  [unwired: 2 in, 2 out]
                              }
                            }
                          }
                        }
                      }
                    }
                  }
                  frame #2 {
                    # "Updates the Cell Status; clears cur SUP cell;  grays out\nSetup button if active GCD cell and current selected cell\nare the same"
                    n323 = global read "Global ER2007.vi" "New GCD Status"() -> (w747:bool)
                    n324 = global read "Global ER2007.vi" "New Sup Status"() -> (w746:bool)
                    n325 = Or(x=w747, y=w746) -> (x .or. y?=w752:bool)
                    n326 = global read "Global ER2007.vi" "SUP Done"() -> (w748:bool)
                    n327 = case shown="True" w752 {
                      tunnel: w747 -> [_ w781]
                      tunnel: w746 -> [_ w780]
                      tunnel: w751 -> [_ _]
                      tunnel: w745 -> [w758 w779]
                      tunnel: [w757 w779] -> w744
                      tunnel: [w756 FALSE] -> w743
                      frame False {
                        # "Updates clock time"
                        n328 = case shown="True" w758 {
                          selector: w758 -> [w761 w763]
                          tunnel: [w761 w765] -> w757
                          tunnel: [FALSE w764] -> w756
                          frame False {
                          }
                          frame True {
                            # "STOP (Exit) in progress"
                            n329 = stacked-sequence {
                              seq-local: [w768 _] -> [_ w775]
                              tunnel: [w767 _] -> w765
                              tunnel: [_ w774] -> w764
                              tunnel: w763 -> [w766 _]
                              frame #0 {
                                n330 = global read "Global ER2007.vi" "STOP Done"() -> (w769:bool)
                                n331 = case shown="False" w769 {
                                tunnel: [FALSE ("STOP Ans") w773] -> w768
                                tunnel: [w770 FALSE] -> w767
                                tunnel: w766 -> [w770 _]
                                frame False {
                                }
                                frame True {
                                n332 = global read "Global ER2007.vi" "STOP Ans"() -> (w773:bool)
                                }
                                }
                              }
                              frame #1 {
                                n333 = case shown="False" w775 {
                                tunnel: [FALSE w777] -> w774
                                frame False {
                                }
                                frame True {
                                w777 = TRUE
                                n334 = global write "Global ER2007.vi" "DAQ Stop"(w777) -> ()
                                n335 = global write "Global ER2007.vi" "GCD Stop"(w777) -> ()
                                }
                                }
                              }
                            }
                          }
                        }
                        n336 = Get Date/Time String(want seconds? (F)=TRUE) -> (time string=→"Clock":string)  [unwired: 2 in, 1 out]
                      }
                      frame True {
                        # "Cell Status File needs to be updated"
                        n337 = stacked-sequence {
                          seq-local: [w783 _] -> [_ w794]
                          tunnel: w781 -> [w784 _]
                          tunnel: w780 -> [w782 _]
                          frame #0 {
                            # "Clear flags &\ngrab initial vals"
                            n338 = case shown="True" w784 {
                              tunnel: [w785 w790] -> w783
                              tunnel: w782 -> [w786 _]
                              frame False {
                                n339 = case shown="False" w786 {
                                tunnel: [w787 w788] -> w785
                                frame False {
                                w787 = 0  # <none>
                                }
                                frame True {
                                n340 = global read "Global ER2007.vi" "SupStatusCell"() -> (w788:i32)
                                n341 = global write "Global ER2007.vi" "New Sup Status"(FALSE ("New Status")) -> ()
                                }
                                }
                              }
                              frame True {
                                n342 = global read "Global ER2007.vi" "GCDStatusCell"() -> (w790:i32)
                                n343 = global write "Global ER2007.vi" "New GCD Status"(FALSE ("New GCD Status")) -> ()
                              }
                            }
                          }
                          frame #1 {
                            # "Updates Cell Status file"
                            n344 = global read "Global ER2007.vi" "Test Info"() -> (w792:T4)
                            n345 = global read "Global ER2007.vi" "Status File Path"() -> (w793:path)
                            n346 = call "Write Cell Status File.vi"("Cell Select"=w794, "Test Info"=w792, "Filepath"=w793) -> ()  [unwired: 8 in, 1 out]
                          }
                        }
                      }
                    }
                    n347 = case shown="True" w748 {
                      tunnel: w750 -> [w753 _]
                      tunnel: [w753 w754] -> w749
                      frame False {
                      }
                      frame True {
                        w754 = 0  # <none>
                        n348 = global write "Global ER2007.vi" "SUP Done"(FALSE ("SUP Done")) -> ()
                      }
                    }
                  }
                }
              }
              frame True {
                # "Something\nchanged"
                n349 = global read "Global ER2007.vi" "Test Info"() -> (w800:T4)
                n350 = case shown="True" w819 {
                  tunnel: w818 -> [w845 _]
                  tunnel: w800 -> [w825 w1022]
                  tunnel: [w844 w1037] -> _
                  tunnel: [w843 w1036] -> w817
                  tunnel: [w842 w1035] -> w816
                  tunnel: [w841 w1034] -> w815
                  tunnel: [w840 w1033] -> w814
                  tunnel: [w839 w1032] -> _
                  tunnel: [w838 w1031] -> _
                  tunnel: [w837 w1030] -> _
                  tunnel: [w836 w1029] -> _
                  tunnel: [w835 w1028] -> w798
                  tunnel: [w834 w1027] -> _
                  tunnel: [w833 w1026] -> w813
                  tunnel: [w832 w1025] -> w811
                  tunnel: [w831 w1024] -> w812
                  tunnel: w810 -> [w830 w1023]
                  tunnel: w809 -> [w829 w1021]
                  tunnel: [w828 w1021] -> w808
                  tunnel: w807 -> [w826 w1020]
                  tunnel: [w827 w1020] -> w806
                  tunnel: [w824 w1019] -> w804
                  tunnel: w803 -> [w823 w1019]
                  tunnel: [w822 w1018] -> w801
                  tunnel: [w821 w1017] -> w797
                  tunnel: [w820 w1016] -> w799
                  frame False {
                    n351 = case shown="False" w845 {
                      tunnel: [w868 w1009] -> w844
                      tunnel: [w851 w1008] -> w843
                      tunnel: [w852 w1007] -> w842
                      tunnel: [w853 w1006] -> w841
                      tunnel: [w854 w1005] -> w840
                      tunnel: [w856 w1004] -> w839
                      tunnel: [w857 w1003] -> w838
                      tunnel: [w858 w1002] -> w837
                      tunnel: [w859 w1001] -> w836
                      tunnel: [w860 w983] -> w835
                      tunnel: [w861 w1000] -> w834
                      tunnel: [w862 w999] -> w833
                      tunnel: [w867 w995] -> w832
                      tunnel: [w855 w996] -> w831
                      tunnel: w830 -> [w866 w995]
                      tunnel: w829 -> [w865 w993]
                      tunnel: [w865 w994] -> w828
                      tunnel: [w863 w991] -> w827
                      tunnel: w826 -> [w864 w991]
                      tunnel: w825 -> [w850 w990]
                      tunnel: [w849 w989] -> w824
                      tunnel: w823 -> [_ w989]
                      tunnel: [w848 TRUE] -> w822
                      tunnel: [w847 w984] -> w821
                      tunnel: [w846 w982] -> w820
                      frame False {
                        n352 = stacked-sequence {
                          seq-local: [w875 _ _] -> [_ w897 _]
                          seq-local: [w874 _ _] -> [_ w900 _]
                          seq-local: [w873 _ _] -> [_ w899 _]
                          seq-local: [w870 _ _] -> [_ w898 _]
                          tunnel: [_ w930 _] -> w868
                          tunnel: [_ w928 _] -> w867
                          tunnel: w866 -> [_ w927 _]
                          tunnel: w864 -> [_ w926 _]
                          tunnel: [_ w925 _] -> w863
                          tunnel: [_ w913 _] -> w862
                          tunnel: [_ w912 _] -> w861
                          tunnel: [_ w911 _] -> w860
                          tunnel: [_ w910 _] -> w859
                          tunnel: [_ w909 _] -> w858
                          tunnel: [_ w908 _] -> w857
                          tunnel: [_ w907 _] -> w856
                          tunnel: [_ w906 _] -> w855
                          tunnel: [_ w905 _] -> w854
                          tunnel: [_ w904 _] -> w853
                          tunnel: [_ w903 _] -> w852
                          tunnel: [_ w902 _] -> w851
                          tunnel: w850 -> [w872 _ _]
                          tunnel: [_ _ w977] -> w849
                          tunnel: [_ _ TRUE] -> w848
                          tunnel: [_ w895 _] -> w847
                          tunnel: [_ w894 _] -> w846
                          frame #0 {
                            # "Updates Busy Captions"
                            # "New Setup"
                            n353 = global read "Global ER2007.vi" "SetupCell"() -> (w871:i32)
                            n354 = global read "Global ER2007.vi" "No Galil"() -> (w869:bool[])
                            n355 = Unbundle By Name(w872) -> ("Cell Data"=w877:T5)
                            n356 = Decrement(x=w871) -> (x-1=w870:i32)
                            n357 = for {
                              tunnel: w869 -> [w880] mode=indexing
                              i -> [w883]
                              n358 = Select(t="Manual", s=w880, f="VPA") -> (s? t:f=w879:string)
                              n359 = case shown="2" w883 {
                                tunnel: w879 -> [_ w884 w885 w886 w887 w888]
                                frame 0, Default {
                                }
                                frame 1 {
                                n360 = property on="C1-Status" class="Bool (strict)"("Caption.Text"=w884) -> ()  [unwired: 2 in, 2 out]
                                }
                                frame 2 {
                                n361 = property on="C2-Status" class="Bool (strict)"("Caption.Text"=w885) -> ()  [unwired: 2 in, 2 out]
                                }
                                frame 3 {
                                n362 = property on="C3-Status" class="Bool (strict)"("Caption.Text"=w886) -> ()  [unwired: 2 in, 2 out]
                                }
                                frame 4 {
                                n363 = property on="C4-Status" class="Bool (strict)"("Caption.Text"=w887) -> ()  [unwired: 2 in, 2 out]
                                }
                                frame 5 {
                                n364 = property on="C5-Status" class="Bool (strict)"("Caption.Text"=w888) -> ()  [unwired: 2 in, 2 out]
                                }
                              }
                            }
                            n365 = Index Array(array=w877, index=w870) -> (element=w878:T6)
                            n366 = Unbundle By Name(w878) -> ("Next Time"=w875:dbl, "Sample #"=w874:string, "Cell Status"=w876:enum16{"Inactive", "Setup", "Active", "Done"})
                            n367 = case shown="\"Active\"" w876 {
                              tunnel: [FALSE TRUE] -> w873
                              frame "Inactive", Default {
                              }
                              frame "Active" {
                              }
                            }
                          }
                          frame #1 {
                            # "New Setup"
                            n368 = global read "Global ER2007.vi" "SUP Cleared"() -> (w896:bool)
                            n369 = case shown="True" w896 {
                              frame False {
                              }
                              frame True {
                                n370 = global write "Global ER2007.vi" "SUP Cleared"(FALSE ("SUP Cleared")) -> ()
                              }
                            }
                            n371 = local read item#-1() -> (w929)
                            n372 = Replace Array Subset(array=w927, new element=w899, index=w898) -> (w928:bool[])
                            n373 = Replace Array Subset(array=w929, new element=w900, index=w898) -> (w930:string[])
                            n374 = local read "ER 1-2"() -> (w924:dbl[])
                            n375 = local read "ER 2-3"() -> (w921:dbl[])
                            n376 = local read "ER 1-3"() -> (w923:dbl[])
                            n377 = local read "ER 1-4"() -> (w922:dbl[])
                            n378 = local read item#-1() -> (w893)
                            n379 = local read item#-1() -> (w914)
                            n380 = local read item#-1() -> (w917)
                            n381 = local read item#-1() -> (w892)
                            n382 = local read item#-1() -> (w891)
                            n383 = Replace Array Subset(array=w926, new element=w897, index=w898) -> (w925:dbl[])
                            n384 = local read "F 2-3"() -> (w920:dbl[])
                            n385 = local read item#-1() -> (w916)
                            n386 = local read item#-1() -> (w919)
                            n387 = local read item#-1() -> (w918)
                            n388 = local read item#-1() -> (w915)
                            n389 = case shown="False" w896 {
                              tunnel: w924 -> [w945 w975]
                              tunnel: w923 -> [w944 w970]
                              tunnel: w922 -> [w943 w969]
                              tunnel: w921 -> [w942 w968]
                              tunnel: w920 -> [w941 w967]
                              tunnel: w919 -> [w940 w959]
                              tunnel: w918 -> [w939 w958]
                              tunnel: w917 -> [w938 w957]
                              tunnel: w916 -> [w937 w956]
                              tunnel: w892 -> [w936 w955]
                              tunnel: w915 -> [w935 w954]
                              tunnel: w914 -> [w934 w953]
                              tunnel: [w934 w966] -> w913
                              tunnel: [w935 w965] -> w912
                              tunnel: [w936 w964] -> w911
                              tunnel: [w937 w963] -> w910
                              tunnel: [w938 w962] -> w909
                              tunnel: [w939 w961] -> w908
                              tunnel: [w940 w960] -> w907
                              tunnel: [w941 w971] -> w906
                              tunnel: [w942 w972] -> w905
                              tunnel: [w943 w973] -> w904
                              tunnel: [w944 w974] -> w903
                              tunnel: [w945 w976] -> w902
                              tunnel: w898 -> [_ w946]
                              tunnel: timestamp(0 s since 1904-01-01) ("*(type *) &x") -> [_ w952]
                              tunnel: [w933 w951] -> w895
                              tunnel: w891 -> [w933 w950]
                              tunnel: [w932 w947] -> w894
                              tunnel: w893 -> [w932 w948]
                              frame False {
                              }
                              frame True {
                                w949 = 0.0 ("new element/subarray")
                                n390 = Replace Array Subset(array=w955, new element=w949, index=w946) -> (w964:dbl[])
                                n391 = Replace Array Subset(array=w953, new element=w949, index=w946) -> (w966:dbl[])
                                n392 = Replace Array Subset(array=w948, new element=w949, index=w946) -> (w947:dbl[])
                                n393 = Replace Array Subset(array=w970, new element=w949, index=w946) -> (w974:dbl[])
                                n394 = Replace Array Subset(array=w968, new element=w949, index=w946) -> (w972:dbl[])
                                n395 = Replace Array Subset(array=w959, new element=w949, index=w946) -> (w960:dbl[])
                                n396 = Replace Array Subset(array=w957, new element=w949, index=w946) -> (w962:dbl[])
                                n397 = Replace Array Subset(array=w954, new element=w952, index=w946) -> (w965:timestamp[])
                                n398 = Replace Array Subset(array=w975, new element=w949, index=w946) -> (w976:dbl[])
                                n399 = Replace Array Subset(array=w969, new element=w949, index=w946) -> (w973:dbl[])
                                n400 = Replace Array Subset(array=w967, new element=w949, index=w946) -> (w971:dbl[])
                                n401 = Replace Array Subset(array=w958, new element=w949, index=w946) -> (w961:dbl[])
                                n402 = Replace Array Subset(array=w956, new element=w949, index=w946) -> (w963:dbl[])
                                n403 = Replace Array Subset(array=w950, new element=w949, index=w946) -> (w951:dbl[])
                              }
                            }
                          }
                          frame #2 {
                            w977 = 0  # <none>
                            n404 = global write "Global ER2007.vi" "New Setup"(FALSE ("New Setup")) -> ()
                          }
                        }
                      }
                      frame True {
                        # "asserts the TakePt flag"
                        # "Take pt - new volume"
                        n405 = global read "Global ER2007.vi" "TakePtCell"() -> (w981:i32)
                        n406 = local read item#-1() -> (w998)
                        n407 = global write "Global ER2007.vi" "TakePt"(FALSE ("New Vol")) -> ()
                        n408 = Unbundle By Name(w990) -> ("Cell Data"=w1010:T5)
                        n409 = Decrement(x=w981) -> (x-1=w980:i32)
                        n410 = Index Array(array=w1010, index=w980) -> (element=w997:T6)
                        n411 = Unbundle By Name(w997) -> ("Last Pore Vol"=w985:dbl)
                        n412 = case shown="False" "Defeated" {
                          tunnel: [w1011 w1015] -> w982
                          tunnel: w998 -> [w1011 w1014]
                          tunnel: w985 -> [_ w1013]
                          tunnel: w980 -> [_ w1012]
                          frame False {
                          }
                          frame True {
                            n413 = Replace Array Subset(array=w1014, new element=w1013, index=w1012) -> (w1015:dbl[])
                          }
                        }
                        n414 = Replace Array Subset(array=w993, new element=TRUE, index=w980) -> (w994:bool[])
                        n415 = local read item#-1() -> (w1000)
                        n416 = local read "ER 1-2"() -> (w1008:dbl[])
                        n417 = local read "ER 2-3"() -> (w1005:dbl[])
                        n418 = local read "ER 1-3"() -> (w1007:dbl[])
                        n419 = local read "ER 1-4"() -> (w1006:dbl[])
                        n420 = local read "F 2-3"() -> (w996:dbl[])
                        n421 = local read item#-1() -> (w999)
                        n422 = local read item#-1() -> (w1004)
                        n423 = local read item#-1() -> (w1002)
                        n424 = local read item#-1() -> (w1003)
                        n425 = local read item#-1() -> (w983)
                        n426 = local read item#-1() -> (w984)
                        n427 = local read item#-1() -> (w1009)
                        n428 = local read item#-1() -> (w1001)
                      }
                    }
                  }
                  frame True {
                    # "New\ndata"
                    n429 = stacked-sequence {
                      seq-local: [w1038 _ _] -> [_ w1047 w1133]
                      seq-local: [w1041 _ _] -> [_ w1061 _]
                      seq-local: [w1040 _ _] -> [_ w1046 w1138]
                      tunnel: w1022 -> [w1043 _ _]
                      tunnel: [_ w1060 _] -> w1037
                      tunnel: [_ w1058 _] -> w1036
                      tunnel: [_ w1057 _] -> w1035
                      tunnel: [_ w1055 _] -> w1034
                      tunnel: [_ w1054 _] -> w1033
                      tunnel: [_ w1052 _] -> w1032
                      tunnel: [_ w1051 _] -> w1031
                      tunnel: [_ w1050 _] -> w1030
                      tunnel: [_ w1049 _] -> w1029
                      tunnel: [_ w1048 _] -> w1028
                      tunnel: [_ w1059 _] -> w1027
                      tunnel: [_ w1056 _] -> w1026
                      tunnel: [_ w1062 _] -> w1025
                      tunnel: [_ w1053 _] -> w1024
                      tunnel: w1023 -> [_ w1062 _]
                      tunnel: [_ _ TRUE] -> w1018
                      tunnel: [_ w1045 _] -> w1017
                      tunnel: [_ w1044 _] -> w1016
                      frame #0 {
                        n430 = global read "Global ER2007.vi" "GCD Err"() -> (w1040:bool)
                        n431 = global read "Global ER2007.vi" "DataCell"() -> (w1039:i32)
                        n432 = Unbundle By Name(w1043) -> ("Cell Data"=w1042:T5)  [unwired: 1 out]
                        n433 = Decrement(x=w1039) -> (x-1=w1038:i32)
                        n434 = Index Array(array=w1042, index=w1038) -> (element=w1041:T6)
                      }
                      frame #1 {
                        n435 = case shown="False" w1046 {
                          tunnel: w1061 -> [w1117 _]
                          tunnel: [w1115 w1132] -> w1060
                          tunnel: [w1069 w1122] -> w1059
                          tunnel: [w1106 w1131] -> w1058
                          tunnel: [w1101 w1130] -> w1057
                          tunnel: [w1098 w1121] -> w1056
                          tunnel: [w1096 w1129] -> w1055
                          tunnel: [w1092 w1128] -> w1054
                          tunnel: [w1090 w1127] -> w1053
                          tunnel: [w1088 w1126] -> w1052
                          tunnel: [w1086 w1125] -> w1051
                          tunnel: [w1080 w1124] -> w1050
                          tunnel: [w1079 w1123] -> w1049
                          tunnel: [w1077 w1120] -> w1048
                          tunnel: w1047 -> [w1068 _]
                          tunnel: [w1071 w1119] -> w1045
                          tunnel: [w1067 w1118] -> w1044
                          frame False {
                            # "No error - update data"
                            n436 = Unbundle By Name(w1117) -> ("Sample #"=w1104:string, "Start Time"=w1073:dbl, "CurData"=w1109:dbl[][])
                            n437 = Get Date/Time In Seconds() -> (seconds since 1Jan1904=w1112:timestamp)
                            n438 = local read item#-1() -> (w1113)
                            n439 = local read item#-1() -> (w1097)
                            n440 = Index Array(array=w1109, index (col)=0 ("disabled index (col)")) -> (element=w1111:dbl[])  [unwired: 1 in]
                            n441 = Array Size(array=w1111) -> (size(s)=w1110:i32)
                            n442 = call "Sample Timer Functions.vi"("Start Time"=w1073) -> ("Elapsed Hours"=w1072:dbl)  [unwired: 5 in, 5 out]
                            n443 = Decrement(x=w1110) -> (x-1=w1103:i32)
                            n444 = Index Array(array=w1109, index (row)=w1103) -> (element=w1108:dbl[])  [unwired: 1 in]
                            n445 = Replace Array Subset(array=w1113, new element=w1112, index=w1068) -> (w1069:timestamp[])
                            n446 = Index Array(array=w1108, index #1=1 ("index")) -> (element #1=w1102:dbl, element #2=w1099:dbl, element #3=w1094:dbl, element #4=w1091:dbl, element #5=w1084:dbl, element #6=w1083:dbl, element #7=w1082:dbl, element #8=w1076:dbl, element #9=w1075:dbl, element #10=w1074:dbl, element #11=w1070:dbl, element #12=w1066:dbl)  [unwired: 11 in]
                            n447 = Replace Array Subset(array=w1097, new element=w1072, index=w1068) -> (w1098:dbl[])
                            n448 = local read "ER 1-2"() -> (w1105:dbl[])
                            n449 = local read "ER 1-4"() -> (w1095:dbl[])
                            n450 = local read "ER 2-3"() -> (w1093:dbl[])
                            n451 = local read "ER 1-3"() -> (w1100:dbl[])
                            n452 = local read "F 2-3"() -> (w1089:dbl[])
                            n453 = local read item#-1() -> (w1087)
                            n454 = local read item#-1() -> (w1085)
                            n455 = local read item#-1() -> (w1081)
                            n456 = local read item#-1() -> (w1078)
                            n457 = local read item#-1() -> (w1064)
                            n458 = local read item#-1() -> (w1065)
                            n459 = local read item#-1() -> (w1063)
                            n460 = local read item#-1() -> (w1116)
                            n461 = Replace Array Subset(array=w1089, new element=w1084, index=w1068) -> (w1090:dbl[])
                            n462 = Replace Array Subset(array=w1105, new element=w1102, index=w1068) -> (w1106:dbl[])
                            n463 = Replace Array Subset(array=w1085, new element=w1082, index=w1068) -> (w1086:dbl[])
                            n464 = Replace Array Subset(array=w1095, new element=w1094, index=w1068) -> (w1096:dbl[])
                            n465 = Replace Array Subset(array=w1064, new element=w1070, index=w1068) -> (w1071:dbl[])
                            n466 = Replace Array Subset(array=w1078, new element=w1075, index=w1068) -> (w1079:dbl[])
                            n467 = Replace Array Subset(array=w1063, new element=w1066, index=w1068) -> (w1067:dbl[])
                            n468 = Replace Array Subset(array=w1116, new element=w1104, index=w1068) -> (w1115:string[])
                            n469 = Replace Array Subset(array=w1100, new element=w1099, index=w1068) -> (w1101:dbl[])
                            n470 = Replace Array Subset(array=w1093, new element=w1091, index=w1068) -> (w1092:dbl[])
                            n471 = Replace Array Subset(array=w1087, new element=w1083, index=w1068) -> (w1088:dbl[])
                            n472 = Replace Array Subset(array=w1081, new element=w1076, index=w1068) -> (w1080:dbl[])
                            n473 = Replace Array Subset(array=w1065, new element=w1074, index=w1068) -> (w1077:dbl[])
                          }
                          frame True {
                            # "GCD error - don't update"
                            n474 = local read item#-1() -> (w1121)
                            n475 = local read "ER 1-2"() -> (w1131:dbl[])
                            n476 = local read "ER 2-3"() -> (w1128:dbl[])
                            n477 = local read "ER 1-3"() -> (w1130:dbl[])
                            n478 = local read "ER 1-4"() -> (w1129:dbl[])
                            n479 = local read item#-1() -> (w1120)
                            n480 = local read item#-1() -> (w1118)
                            n481 = local read item#-1() -> (w1124)
                            n482 = local read item#-1() -> (w1132)
                            n483 = local read item#-1() -> (w1119)
                            n484 = local read "F 2-3"() -> (w1127:dbl[])
                            n485 = local read item#-1() -> (w1123)
                            n486 = local read item#-1() -> (w1126)
                            n487 = local read item#-1() -> (w1125)
                            n488 = local read item#-1() -> (w1122)
                          }
                        }
                      }
                      frame #2 {
                        # "Clears flags, updates selected cell status"
                        n489 = case shown="True" w1138 {
                          tunnel: [FALSE ("C1-Status") TRUE ("C1-Status")] -> w1137
                          tunnel: [w1149 w1151] -> w1136
                          frame False {
                            w1149 = cluster{u32, u32}[] [{1985280, 1985280}, {6618880, 6618880}, {1985280, 1985280}, {6618880, 6618880}]  # Busy Colors
                            # "No error"
                          }
                          frame True {
                            w1151 = cluster{u32, u32}[] [{1985280, 1985280}, {15670784, 15670784}, {1985280, 1985280}, {7802624, 7802624}]  # Error Colors
                            # "GCD error"
                          }
                        }
                        n490 = global write "Global ER2007.vi" "New Data"(FALSE ("New Data")) -> ()
                        n491 = case shown="1" w1133 {
                          tunnel: w1137 -> [w1140 w1142 w1144 w1146 w1148]
                          tunnel: w1136 -> [w1139 w1141 w1143 w1145 w1147]
                          frame 0, Default {
                            n492 = property on="C1-Status" class="Bool (strict)"("Value"=w1140, "Colors [4]"=w1139) -> ()  [unwired: 2 in, 2 out]
                          }
                          frame 1 {
                            n493 = property on="C2-Status" class="Bool (strict)"("Value"=w1142, "Colors [4]"=w1141) -> ()  [unwired: 2 in, 2 out]
                          }
                          frame 2 {
                            n494 = property on="C3-Status" class="Bool (strict)"("Value"=w1144, "Colors [4]"=w1143) -> ()  [unwired: 2 in, 2 out]
                          }
                          frame 3 {
                            n495 = property on="C4-Status" class="Bool (strict)"("Value"=w1146, "Colors [4]"=w1145) -> ()  [unwired: 2 in, 2 out]
                          }
                          frame 4 {
                            n496 = property on="C5-Status" class="Bool (strict)"("Value"=w1148, "Colors [4]"=w1147) -> ()  [unwired: 2 in, 2 out]
                          }
                        }
                      }
                    }
                  }
                }
                "ER 1-2" <- w817
                "ER 1-3" <- w816
                "ER 1-4" <- w815
                "ER 2-3" <- w814
                "F 2-3" <- w812
              }
            }
            "SelCell" <- w492
            "SetupCell" <- w491
          }
          event #1 (no event record) {
            # "Cell Selects chgd"
            n497 = event-data() -> ("NewVal"=w1161)  [unwired: 1 in]
            n498 = case shown="\"CS 1\", Default" w1161 {
              selector: w1161 -> [_ w1166]
              tunnel: w1158 -> [_ _]
              tunnel: [w1164 w1165] -> w1157
              frame "No Selection" {
                w1164 = 0  # <none>
              }
              frame "CS 1", Default {
                n499 = case shown="\"No Selection\", Default" w1166 {
                  tunnel: [w1167 1 2 3 4 5] -> w1165
                  frame "No Selection", Default {
                    w1167 = 0  # <none>
                  }
                  frame "CS 1" {
                  }
                  frame "CS 2" {
                  }
                  frame "CS 3" {
                  }
                  frame "CS 4" {
                  }
                  frame "CS 5" {
                  }
                }
              }
            }
          }
          event "TakePt": Value Change {
            # "TakePt chgd"
            n500 = event-data() -> ()  [unwired: 1 in, 1 out]
            n501 = stacked-sequence {
              tunnel: w1181 -> [w1184 _]
              frame #0 {
                # "Loads the Cell #"
                n502 = case shown="\"No Selection\", Default" w1184 {
                  tunnel: [0 1 ("Selected Radio Cell") 2 ("Selected Radio Cell") 3 ("Selected Radio Cell") 4 ("Selected Radio Cell") 5 ("Selected Radio Cell")] -> w1183
                  frame "No Selection", Default {
                  }
                  frame "CS 1" {
                  }
                  frame "CS 2" {
                  }
                  frame "CS 3" {
                  }
                  frame "CS 4" {
                  }
                  frame "CS 5" {
                  }
                }
                n503 = global write "Global ER2007.vi" "TakePtCell"(w1183) -> ()
              }
              frame #1 {
                # "Runs the popup panel vi"
                n504 = Open VI Reference(vi path=path "ER2007 Take Data Popup Panel.vi") -> (vi reference=w1198:refnum<vi>, error out=w1197:errorcluster)  [unwired: 5 in]
                n505 = property class="VI"(reference=w1198, error in=w1197, "Front Panel Window:Open"=TRUE) -> (reference out=w1195:refnum<vi>, error out=w1194:errorcluster)
                n506 = invoke class="VI" method="Run VI"(reference=w1195, error in=w1194, "Wait until done"=FALSE, "Auto Dispose Ref"=TRUE) -> (error out=w1191:errorcluster)  [unwired: 1 in, 4 out]
                n507 = call <vilib>:"Simple Error Handler.vi"("error in (no error)"=w1191) -> ()  [unwired: 4 in, 5 out]
              }
            }
          }
          event "Setup": Value Change {
            # "Setup"
            n508 = event-data() -> ()  [unwired: 1 in, 1 out]
            n509 = stacked-sequence {
              tunnel: w1208 -> [w1211 _]
              tunnel: [w1210 _] -> w1204
              frame #0 {
                n510 = case shown="\"No Selection\", Default" w1211 {
                  tunnel: [0 1 ("Selected Radio Cell") 2 ("Selected Radio Cell") 3 ("Selected Radio Cell") 4 ("Selected Radio Cell") 5 ("Selected Radio Cell")] -> w1210
                  frame "No Selection", Default {
                  }
                  frame "CS 1" {
                  }
                  frame "CS 2" {
                  }
                  frame "CS 3" {
                  }
                  frame "CS 4" {
                  }
                  frame "CS 5" {
                  }
                }
                n511 = global write "Global ER2007.vi" "New Setup"(FALSE ("New Setup")) -> ()
                n512 = global write "Global ER2007.vi" "SetupCell"(w1210) -> ()
              }
              frame #1 {
                # "Launches Test Def Panel (Setup)"
                n513 = Open VI Reference(vi path=path "ER2007 Test Definition Panel.vi") -> (vi reference=w1226:refnum<vi>, error out=w1225:errorcluster)  [unwired: 5 in]
                n514 = property class="VI"(reference=w1226, error in=w1225, "Front Panel Window:Open"=TRUE) -> (reference out=w1223:refnum<vi>, error out=w1222:errorcluster)
                n515 = invoke class="VI" method="Run VI"(reference=w1223, error in=w1222, "Wait until done"=FALSE, "Auto Dispose Ref"=TRUE) -> (error out=w1219:errorcluster)  [unwired: 1 in, 4 out]
                n516 = call <vilib>:"Simple Error Handler.vi"("error in (no error)"=w1219) -> ()  [unwired: 4 in, 5 out]
              }
            }
          }
          event "History": Value Change {
            # "History"
            n517 = event-data() -> ()  [unwired: 1 in, 1 out]
            n518 = stacked-sequence {
              tunnel: w1236 -> [w1239 _]
              frame #0 {
                n519 = case shown="\"No Selection\", Default" w1239 {
                  tunnel: [0 1 ("Selected Radio Cell") 2 ("Selected Radio Cell") 3 ("Selected Radio Cell") 4 ("Selected Radio Cell") 5 ("Selected Radio Cell")] -> w1238
                  frame "No Selection", Default {
                  }
                  frame "CS 1" {
                  }
                  frame "CS 2" {
                  }
                  frame "CS 3" {
                  }
                  frame "CS 4" {
                  }
                  frame "CS 5" {
                  }
                }
                n520 = global write "Global ER2007.vi" "SetupCell"(w1238) -> ()
              }
              frame #1 {
                n521 = Open VI Reference(vi path=path "ER2007 Data History Panel.vi") -> (vi reference=w1253:refnum<vi>, error out=w1252:errorcluster)  [unwired: 5 in]
                n522 = property class="VI"(reference=w1253, error in=w1252, "Front Panel Window:Open"=TRUE) -> (reference out=w1250:refnum<vi>, error out=w1249:errorcluster)
                n523 = invoke class="VI" method="Run VI"(reference=w1250, error in=w1249, "Wait until done"=FALSE, "Auto Dispose Ref"=TRUE) -> (error out=w1246:errorcluster)  [unwired: 1 in, 4 out]
                n524 = call <vilib>:"Simple Error Handler.vi"("error in (no error)"=w1246) -> ()  [unwired: 4 in, 5 out]
              }
            }
          }
          event "CurVals": Value Change {
            # "Current values"
            n525 = event-data() -> ()  [unwired: 1 in, 1 out]
            n526 = Open VI Reference(vi path=path "ER2007 Current Values Panel.vi") -> (vi reference=w1270:refnum<vi>, error out=w1269:errorcluster)  [unwired: 5 in]
            n527 = property class="VI"(reference=w1270, error in=w1269, "Front Panel Window:Open"=TRUE) -> (reference out=w1267:refnum<vi>, error out=w1266:errorcluster)
            n528 = invoke class="VI" method="Run VI"(reference=w1267, error in=w1266, "Wait until done"=FALSE, "Auto Dispose Ref"=TRUE) -> (error out=w1263:errorcluster)  [unwired: 1 in, 4 out]
            n529 = call <vilib>:"Simple Error Handler.vi"("error in (no error)"=w1263) -> ()  [unwired: 4 in, 5 out]
          }
          event "Utilities": Value Change {
            # "Utilities"
            n530 = event-data() -> ()  [unwired: 1 in, 1 out]
            n531 = Open VI Reference(vi path=path "ER2007 Password Popup Panel.vi") -> (vi reference=w1291:refnum<vi>, error out=w1290:errorcluster)  [unwired: 5 in]
            n532 = property class="VI"(reference=w1291, error in=w1290, "Front Panel Window:Open"=TRUE) -> (reference out=w1288:refnum<vi>, error out=w1287:errorcluster)
            n533 = invoke class="VI" method="Run VI"(reference=w1288, error in=w1287, "Wait until done"=FALSE, "Auto Dispose Ref"=TRUE) -> (error out=w1284:errorcluster)  [unwired: 1 in, 4 out]
            n534 = call <vilib>:"Simple Error Handler.vi"("error in (no error)"=w1284) -> ()  [unwired: 4 in, 5 out]
          }
          event "Reset DAQ": Value Change {
            # "Reset DAQ"
            n535 = event-data() -> ("NewVal"=w1295:bool)  [unwired: 1 in]
            n536 = case shown="True" w1295 {
              frame False {
              }
              frame True {
                n537 = global write "Global ER2007.vi" "DAQ Init"(TRUE) -> ()
              }
            }
          }
          event "Stop": Value Change {
            # "Stop"
            n538 = event-data() -> ()  [unwired: 1 in, 1 out]
            n539 = stacked-sequence {
              frame #0 {
                n540 = global write "Global ER2007.vi" "STOP Done"(FALSE ("STOP Done")) -> ()
              }
              frame #1 {
                n541 = Open VI Reference(vi path=path "ER2007 Are You Sure Popup Panel.vi") -> (vi reference=w1323:refnum<vi>, error out=w1322:errorcluster)  [unwired: 5 in]
                n542 = property class="VI"(reference=w1323, error in=w1322, "Front Panel Window:Open"=TRUE) -> (reference out=w1320:refnum<vi>, error out=w1319:errorcluster)
                n543 = invoke class="VI" method="Run VI"(reference=w1320, error in=w1319, "Wait until done"=FALSE, "Auto Dispose Ref"=TRUE) -> (error out=w1316:errorcluster)  [unwired: 1 in, 4 out]
                n544 = call <vilib>:"Simple Error Handler.vi"("error in (no error)"=w1316) -> ()  [unwired: 4 in, 5 out]
              }
            }
          }
        }
        "Status" <- w472
        "Refresh" <- w460
        "Schd Times" <- w468
        "GCDCell" <- w464
      }
    }
    frame #2 {
      # "Cleanup and shutdown"
      n545 = stacked-sequence {
        tunnel: w1325 -> [w1329 _ _]
        frame #0 {
          w1326 = FALSE ("Visible")
          w1328 = TRUE  # Stop
          w1331 = FALSE ("C1-Status")
          w1327 = FALSE ("A/D Run")
          w1332 = u8 0 ("Disabled")
          # "Clears variables and properties"
          n546 = global write "Global ER2007.vi" "SysRun"(FALSE ("SysRun")) -> ()
          n547 = local write "Status"(bool[] [FALSE, FALSE, FALSE, FALSE, FALSE] ("Status")) -> ()
          n548 = property on="TakePt" class="Bool"("Disabled"=w1332) -> ()  [unwired: 2 in, 2 out]
          n549 = property on="System Error" class="Bool (strict)"("Visible"=w1326) -> ()  [unwired: 2 in, 2 out]
          n550 = local write "DAQ Run"(w1327) -> ()
          n551 = call "Sample Request Control.vi"("SimOn"=w1329, "Stop"=w1328) -> ()  [unwired: 12 in, 6 out]
          n552 = local write item#-1(T1."No Selection" ("Radio Cell Selects")) -> ()
          n553 = property on="Setup" class="Bool"("Disabled"=w1332) -> ()  [unwired: 2 in, 2 out]
          n554 = property on="Reset DAQ" class="Bool"("Visible"=w1326) -> ()  [unwired: 2 in, 2 out]
          n555 = local write "A/D Err"(w1327) -> ()
          n556 = property on="History" class="Bool"("Disabled"=w1332) -> ()  [unwired: 2 in, 2 out]
          n557 = local write "GCD Busy"(w1327) -> ()
          n558 = property on="CurVals" class="Bool"("Disabled"=w1332) -> ()  [unwired: 2 in, 2 out]
          n559 = local write "GCD Err"(w1327) -> ()
          n560 = local write "VPA Err"(w1327) -> ()
          "C1-Status" <- w1331
          "C2-Status" <- w1331
          "C3-Status" <- w1331
          "C4-Status" <- w1331
          "C5-Status" <- w1331
        }
        frame #1 {
          # "Waits for Get Cell Data to Stop"
          n561 = Get Date/Time In Seconds() -> (seconds since 1Jan1904=w1336:timestamp)
          n562 = To Double Precision Float(number=w1336) -> (double precision float=w1335:dbl)
          n563 = while {
            tunnel: w1335 -> [w1342]
            stop <- w1340 continue-if-true
            w1341 = 8.0  # T/O = 8 sec
            n564 = Get Date/Time In Seconds() -> (seconds since 1Jan1904=w1344:timestamp)
            n565 = To Double Precision Float(number=w1344) -> (double precision float=w1343:dbl)
            n566 = Subtract(x=w1343, y=w1342) -> (x-y=w1338:dbl)
            n567 = Wait Until Next ms Multiple(millisecond multiple=u32 300) -> ()  [unwired: 1 out]
            n568 = global read "Global ER2007.vi" "GCD Stop"() -> (w1337:bool)
            n569 = Less?(x=w1338, y=w1341) -> (x < y?=w1339:bool)
            n570 = And(x=w1339, y=w1337) -> (x .and. y?=w1340:bool)
          }
        }
        frame #2 {
          # "Exits to LabVIEW or Windows"
          n571 = global read "Global ER2007.vi" "Quit2LV"() -> (w1346:bool)
          n572 = Not(x=w1346) -> (.not. x?=w1347:bool)
          n573 = Quit LabVIEW(quit? (T)=w1347) -> ()
        }
      }
    }
  }
